vi "Core_Chem_User_Interface_v1.3.vi"() -> ()   [LabVIEW 2014]
uses:
  C:/Program Files (x86)/National Instruments/LabVIEW 2014/examples/Data Communication/Network Streams/Simple Network Streams/support/Network Stream Command.ctl
  <vilib>/dex/Stream Element Allocation Mode.ctl
  <vilib>/Platform/TimedLoop/XDataNode/wakeup.ctl
  <vilib>/Platform/TimedLoop/XDataNode/XDNodeRunTimeDep.lvlib
  <vilib>/Platform/TimedLoop/XDataNode/nitl_modes.ctl
  <vilib>/Platform/TimedLoop/XDataNode/timing_clust.ctl
  <vilib>/platform/TimedLoop/XDataNode/XDataNode.xnode
  <vilib>/Utility/tcp.llb/UDP Multicast Read-Only Open.vi
  <vilib>/FTP/NI_FTP.lvlib
panel:
  out "Create folder error out 2":errorcluster
  out "Network to cRIO live status":bool
  out "Create folder error out":errorcluster
  in  "Confirm Flight Number":bool
  out "PRTAFT_UDP_In":string
  out "TWBOZO01":string
  out "CABOZO01":string
  out "TEIOZO01":string
  out "CHTSOO01":string
  out "CHFGGA01":string
  out "AL52CO01":string
  in  "Flight Number":string
  in  "Tab Control":T1(tab)
  out "FGGA preflight Des 17":string="Preflight - Start minimum 2 hours before take-off\n\n1. Ensure no bags/jackets are stowed on seat backs and behind seats in front of core chemistry rack at all times.\n\n2. Remove inlet covers if applicable.\n\n3. Connect Lilliput mini TFT/LCD VGA cable to FGGA VIDEO (back panel) and PS2 Keyboard/Mouse cables to FGGA Connectors (back panel). TFT/LCD and Keyboard kept in Core Chemistry Dell laptop bag. Connect TFT/LCD AC/DC PSU to 6026-8-98 Amphenol (SSP9) and make 230 Vac CB.\n\n4. Ensure all circuit breakers are pushed in, except 230Vac and 28Vdc, UPS switch off (down) and AL5002 CO Plasma Lamp switch off (down).\n\n5. Wait for aircraft LAN to be up and running before start-up.\n\n6. Check AboutTime has synchronised laptop clock to aircraft timeservers (Filiberto/Gaston).\n\nClick the PowerUp Tab."
  out "FGGA preflight Des 16":string="PowerUp\n\n1.\tSSP9 forward face\tMake 3 CBs\n\n2.\tPWRDIST \t\tMake 230Vac CB Switch UPS On \t[UP]\n                     Make 28Vdc CB\n                     Check 28VDC OK Green Light comes on\n\n3.\tCore Chemistry e-Log\nComplete Core Chemistry e-Log in WordPad (Bnnn_CoreChemLog_v2.1), save on Flight Manager's laptop (192.168.101.180/      flt_folders/Bnnn); Fill in header with date, flight number and your name/initials.\n\n4.\tSAMPUMP\t\t\n - Switch WoW override key (vertical) to check pump starts, and MFM flowrate increase (>20 LPM) under System Overview tab. \n - Switch off WoW override\t\t\t\t [NORM, key horizontal]\n\nClick the 2B Ozone tab if operated, otherwise, click the UDP tab.\n\n\n"
  out "MFM":dbl(graph)
  in  "Ambient = OFF\nCabin = ON":bool
  out "FGGA preflight Des 15":string="2B Ozone Preflight\n\n1.\tSelect either Ambient or Cabin Air mode (default should be OFF for Ambient air mode).\n\n2. Check flowrate is greater than 2000 sccm.\n\nClick the UDP tab."
  out "2B Ozone concentration":dbl(graph)
  out "2B Ozone flow rate":dbl(graph)
  out "2BOzone Event error out":errorcluster
  out "2BOzone command sender error out":errorcluster
  out "FGGA preflight Des 14":string="UDP Preflight\n1. Check all UDP packets are updating.  Unix time increasing by 1 sec (2nd parameter).\n2. Check flight number is correct.\n3. Confirm flight number and check it appears in the UDP packet. "
  in  "name":string="239.1.4.6"
  in  "Port":u16=50001
  out "FGGA":string
  out "CO":string
  out "Ozone":string
  out "Cabin Ozone":string
  out "Ambient Ozone":string
  out "SO2":string
  out "Ozone Zeroing\nTime Remain (sec)":u32
  in  "Ozone Zeroing":bool
  out "TEI49C Sample Flow B":dbl(graph)
  out "TEi49C Concentration":dbl(graph)
  out "TEI49C Sample Flow A":dbl(graph)
  out "FGGA preflight Des 13":string="TEi49C Ozone PRE-FLIGHT - LAST ACTIONS BEFORE SEAT-BELTING DOWN (PRIOR TO ENGINES START)\n\n1. Ozone monitor zeroing\t\t[10 min minimum]\n\n\n2. Check TEi49C zero value and note down value in e-Log. \n"
  out "FGGA preflight Des 12":string="TEi49C Ozone Preflight\n\n1. Check nominal sample flowrate on both channels is ~0.7 LPM."
  out "Ozone Event error out":errorcluster
  out "Ozone command sender error out":errorcluster
  in  "Ozone UDP Time Offset":i32=1
  out "SO2 Flush\nTime Remain (sec)":u32
  out "TEI43i MFC3 Sample Flow":dbl(graph)
  out "TEi43C / TEi43i Concentration":dbl(graph)
  out "TEI43C Sample Flow":dbl(graph)
  out "TEI43i MFC2 Cal Flow":dbl(graph)
  in  "MFC_2 User Set Value":dbl=2.5
  in  "MFC_3 User Set Value":dbl=2.0
  out "SO2 CAL\nTime Remain (sec)":u32
  out "SO2 Cal Flush\nTime Remain (sec)":u32
  in  "SO2 CAL":bool
  out "FGGA preflight Des 11":string="TEi43 SO2 Inflight Calibration"
  in  "SO2 Zeroing":bool
  out "SO2 Zeroing\nTime Remain (sec)":u32
  out "FGGA preflight Des 10":string="TEi43 SO2 PRE-FLIGHT - LAST ACTIONS BEFORE SEAT-BELTING DOWN (PRIOR TO ENGINES START)\n\n1. SO2 monitors zeroing\t\t[10 min minimum]\n\n\n2. Check TEi43i or TEi43C zero value and note down value in e-Log. "
  in  "SO2 Flush":bool
  out "FGGA preflight Des 9":string="TEi43 SO2 Preflight\n\n1. Check nominal sample flowrate is 2.0 LPM.\n\nSO2 calibration gas purge - SO2 calibration cylinder locate at bottom of WAS Gas rack.\n\n2. Check quick connect male body is connected to 'chem 1' gas line.\n\n3. Open cylinder valve 1.\n\n4. Set regulator to deliver at 3 bar.\n\n5. Open regulator valve 3 (anti-clockwise).\n\n6. Close cylinder valve 1.\n\n7. Press SO2 flush button, MFC2 cal flow should increase to 2.5 SLPM.\nMonitor MFC2 flow rate to make sure the reading decreases from 2.5 SLPM to 0.0 SLPM.\nCheck pressure content and delivery guages also reasd zero.\nIf pressure content & delivery guages do NOT read zero, press SO2 flush button again until they do.\n\n8. Quickly open and close cylinder valve 1.\n\n9. Repeat step 7) to 8) three times.\n\n10. Open cylinder valve 1, system is ready.\n "
  in  "eV9 Flush User\nset time (sec)":i32=15
  in  "eV9 flush User\nset time (sec)":i32=60
  in  "eV8 User\nset time (sec)":i32=120
  out "SO2 Event error out":errorcluster
  out "SO2 command sender error out":errorcluster
  in  "SO2 UDP Time Offset":i32=1
  out "CO CAL Status":bool
  in  "CO CAL":bool
  out "FGGA preflight Des 8":string="CO Preflight and Inflight Calibrations\nHold down the CAL button for 2 secs then release, CAL status should then lit up"
  in  "Prepare Gases":bool
  out "FGGA preflight Des 7":string="AL5002 CO Preflight Checks\n\n1.\n\n2. Start CO Vacuum. NB: If there is problem with the software control, use manual override switch [up] on CALDECK front panel\n\n3. CO Checks - charts on the right hand side\n    Lamp Flow Controller ~ 40 ml/min\n    Monochromater Flow Controller ~ 30 ml/min\n    Fluorescence Cell Pressure ~ 7.5 Torr\n\nIf Lamp/Mono flows are low, manual valves (V1 -> V5) may still be shut, or pressure adjusting valves (ALREG1 & 2) have not been set > 2 bar\n\nIf Cell pressure is 10 Torr (max range), check that COPUMP is running and eV7 is opened (CALDECK green LED).\n\n4. Switch Plasma Lamp at the front panel UP\n\nDetector count rate (on 'Raw Signal' or F2 instrument touchscreen) should increase to >=10000 Hz within a minute.  Recycle plasma lamp switch (off/on) if no significant increase in count rate after 10 mins.  CO concentration should increase (100s ppb). \n     \n\n"
  in  "CO Vacuum (eV7)":bool
  out "Raw Signal":dbl(graph)
  out "CO Concentration":dbl(graph)
  out "Fluorsecence Cell Pressure":dbl(graph)
  out "Monochromater Flow":dbl(graph)
  out "Lamp Flow Controller":dbl(graph)
  in  "CO UDP Time Offset":i32=1
  out "CO2 Pressure\nDelivery (PSIA)":dbl(slide) scale=0.0..100.0
  out "Std\nContent (barG)":dbl(slide) scale=0.0..220.0
  out "N2\nContent (barG)":dbl(slide) scale=0.0..220.0
  out "CO2\nContent (barG)":dbl(slide) scale=0.0..170.0
  out "CO Event error out":errorcluster
  out "CO command sender error out":errorcluster
  out "CO Zero":T2(array[cluster])
  out "CO Sensitivity":T3(array[cluster])
  out "Cell temperature":dbl(graph)
  out "Cell pressure":dbl(graph)
  in  "Manual FGGA Pump":bool
  out "CO2":dbl(graph)
  out "CH4":dbl(graph)
  out "H2O":dbl(graph)
  out "WoW Flag":string="0"
  in  "FGGA pump\nsync to WoW":bool
  out "CH4 Dry":dbl(graph)
  out "CO2 Dry":dbl(graph)
  out "MFC1 Cal Flow":dbl(graph)
  out "Flush Target Tank\nTime Remain (sec)":u32
  out "Flush Low Tank\nTime Remain (sec)":u32
  out "Flush High Tank\nTime Remain (sec)":u32
  in  "Flush Target Tank":bool
  in  "Flush Low Tank":bool
  in  "Flush High Tank":bool
  in  "FGGA Restart":bool
  out "FGGA preflight Des 6":string="FGGA Instrument Controls"
  in  "High Cal":bool
  out "High Cal\nFlush Time Remain (sec)":u32
  out "High Cal\nCal Time Remain (sec)":u32
  in  "Low Cal":bool
  in  "Target Cal":bool
  in  "Span Cal - \nHigh Cal, CO Cal, Low Cal":bool
  out "Low Cal\nFlush Time Remain (sec)":u32
  out "Low Cal\nCal Time Remain (sec)":u32
  out "Target Cal\nFlush Time Remain (sec)":u32
  out "Target Cal\nCal Time Remain (sec)":u32
  in  "MFC_1 User Set Value":dbl=3.0
  out "FGGA preflight Des 5":string="FGGA Inflight Calibrations"
  out "FGGA preflight Des 4":string="FGGA Ground Preflight Checks\n\n1. Switch FGGA pump ON\n\n2. Check cavity pressure ~50 Torr\n\n3. Switch FGGA pump OFF\n\n4. Enable FGGA pump sync to WoW\n\n5.. Check Time Synchronisation\n\n6. Check CO2 & CH4 values\n"
  out "FGGA preflight Des 3":string="FGGA CAL Gas Purge\n\nFor each cylinder in gas stowage, check that,\n\n1. V1 Closed\n    V3 Closed\n    V4 Make sure arrow positioned downwards (i.e. flow points to gas line)\n\n2. V3 Open (turn anti-clockwise)\n\n3. Use the button on the right according to the operating cylinder to flush the line. Monitor the MFC flow rate to make sure the reading decreases from 3 to zero. (ie fully flushed). Pressure content & delivery gauges should also read zero.\n\n4. V3 Close (turn clockwise)\n\n5. V1 Open / Close quickly\n         Check delivery pressure gauge is ~ 40 PSI \n         (Use V2 to increase if necessary)\n\n6. Repeat steps 2) to 5) three times\n\n7. V3 Close (turn clockwise)\n\n8. V1 Open, check V2 ~ 40 PSIG\n\n9. V3 Open - System is ready"
  out "FGGA command sender error out":errorcluster
  out "FGGA Event Error out":errorcluster
  in  "FGGA UDP Time Offset":i32=1
  in  "FGGA Shutdown":bool
  in  "Postflight Procedures":bool
  in  "cRIO File IO Stop\n(USB Flash Drive Unmount)":bool
  in  "FTP ASCII Files to Local":bool
  in  "Transfer FGGA Files":bool
  out "FGGA preflight Des 18":string="Postflight\n\n1. Press the cRIO File IO Stop to stop ASCII file recording\nNote: ASCIII file recording will start again once the flight number is confirmed.\n\n2. Press the FTP ASCII File to Local button to transfer ASCII files to flight folder.\n\n\n3. Press the Transfer FGGA Files button to transfer FGGA files to flight folder. \n\n4. Shutdown FGGA.\n\n\n5. View Postflight Procedures."
  out "File List":string[](array[string])
  out "FGGA File Transfer Error out":errorcluster
  out "Move to FM Error out":errorcluster
  out "USB Disk Space Used %":dbl(slide) scale=0.0..100.0
  out "PTP Sync":bool
  out "CPU Total %":dbl(graph)
  out "PRTAFT_DLU":string
  in  "Inst_alm_thresh":i32=220
  in  "3hr_alm_thresh":i32=80
  in  "Simulate Inst Conc":i32
  in  "Simulate 3hr Average Conc":dbl
  in  "Simulate 2B Conc":bool
  in  "Ozone eV6":bool
  in  "Simulate Conc":bool
  in  "8hr TWA Limit":i32=490
  in  "10mins STEL Limit":i32=700
  in  "SO2 Slope":dbl=1.0
  in  "SO2 Offset":dbl
  in  "Simulate TWA Conc":dbl
  in  "Simulate STEL Conc":dbl
  in  "MFC_3\nSLPM Value":dbl=2.0
  in  "MFC_2\nSLPM Value":dbl
  in  "SO2 eV6":bool
  in  "eV8":bool
  in  "eV9":bool
  in  "eV4":bool
  in  "eV3":bool
  in  "MFC_1\nSLPM Value":dbl
  in  "eV2":bool
  in  "eV1":bool
  # "concentration\npmt_volt\nlamp_volt\nlamp_intens\ninternal_temper\nreact_temper\nreact_press\nflow\nflags\nten_min_so2\neight_hr_so2\nten_min_so2_alm\neight_hr_so2_alm\nMFC_2absolute_pres\nMFC_2temperature\nMFC_2volumetic_flow\nMFC_2mass_flow\nMFC_2set_point\nMFC_3_absolute_pres\nMFC_3_temperature\nMFC_3volumetic_flow\nMFC_3mass_flow\nMFC_3set_point\nV6\nV8\nV9\nMFC2_Set_Value\nMFC3_Set_Value"
  # "conc\ntemp\npress\nflow\nthreehr_oz\nInst_alarm\nthreehr_alarm"
  # "ch4\nco2\nh2o\npress_torr\ntemp_c\nfit_flag\nrda_usec\nrdb_usec\nch4_dry\nco2_dry\nMFC_1_absolute_pres\nMFC_1_temperature\nMFC_1volumetic_flow\nMFC_1mass_flow\nMFC_1set_point\nV1\nV2\nV3\nV4\nrestart_FGGA\nFGGA_Pump\nCAL_MFC_1Set_Value"
  # "conc\ntemp\npress\nflow"
  # "conc\nbenchtemp\npress\ncellAint\ncellBint\nFlowA\nFlowB\nlamptemp\nflag\nV6"
  # "conc\ncounts\nsens\nzero\nlampflow\nlamptemp\nmonoflow\nmonotemp\nmonopress\ncellpress\ncalpress\ntemppmt\ncalconc\nerr\ncal_counter\nerr_counter\nCO_vacuum_status\nIn_Cal\nALEG1_press_delivery\nALREG1_press_content\nALREG2_press_content\nALREG3_press_content"
  # "TEi43c"
  # "TEi43i"
  # "SO2 CAL SETTINGS"
  # "SO2 FLUSH SETTING"
  # "FGGA"
  # "2B Ozone"
  # "TEi49C  - Ozone"
  # "TEi43 - SO2"
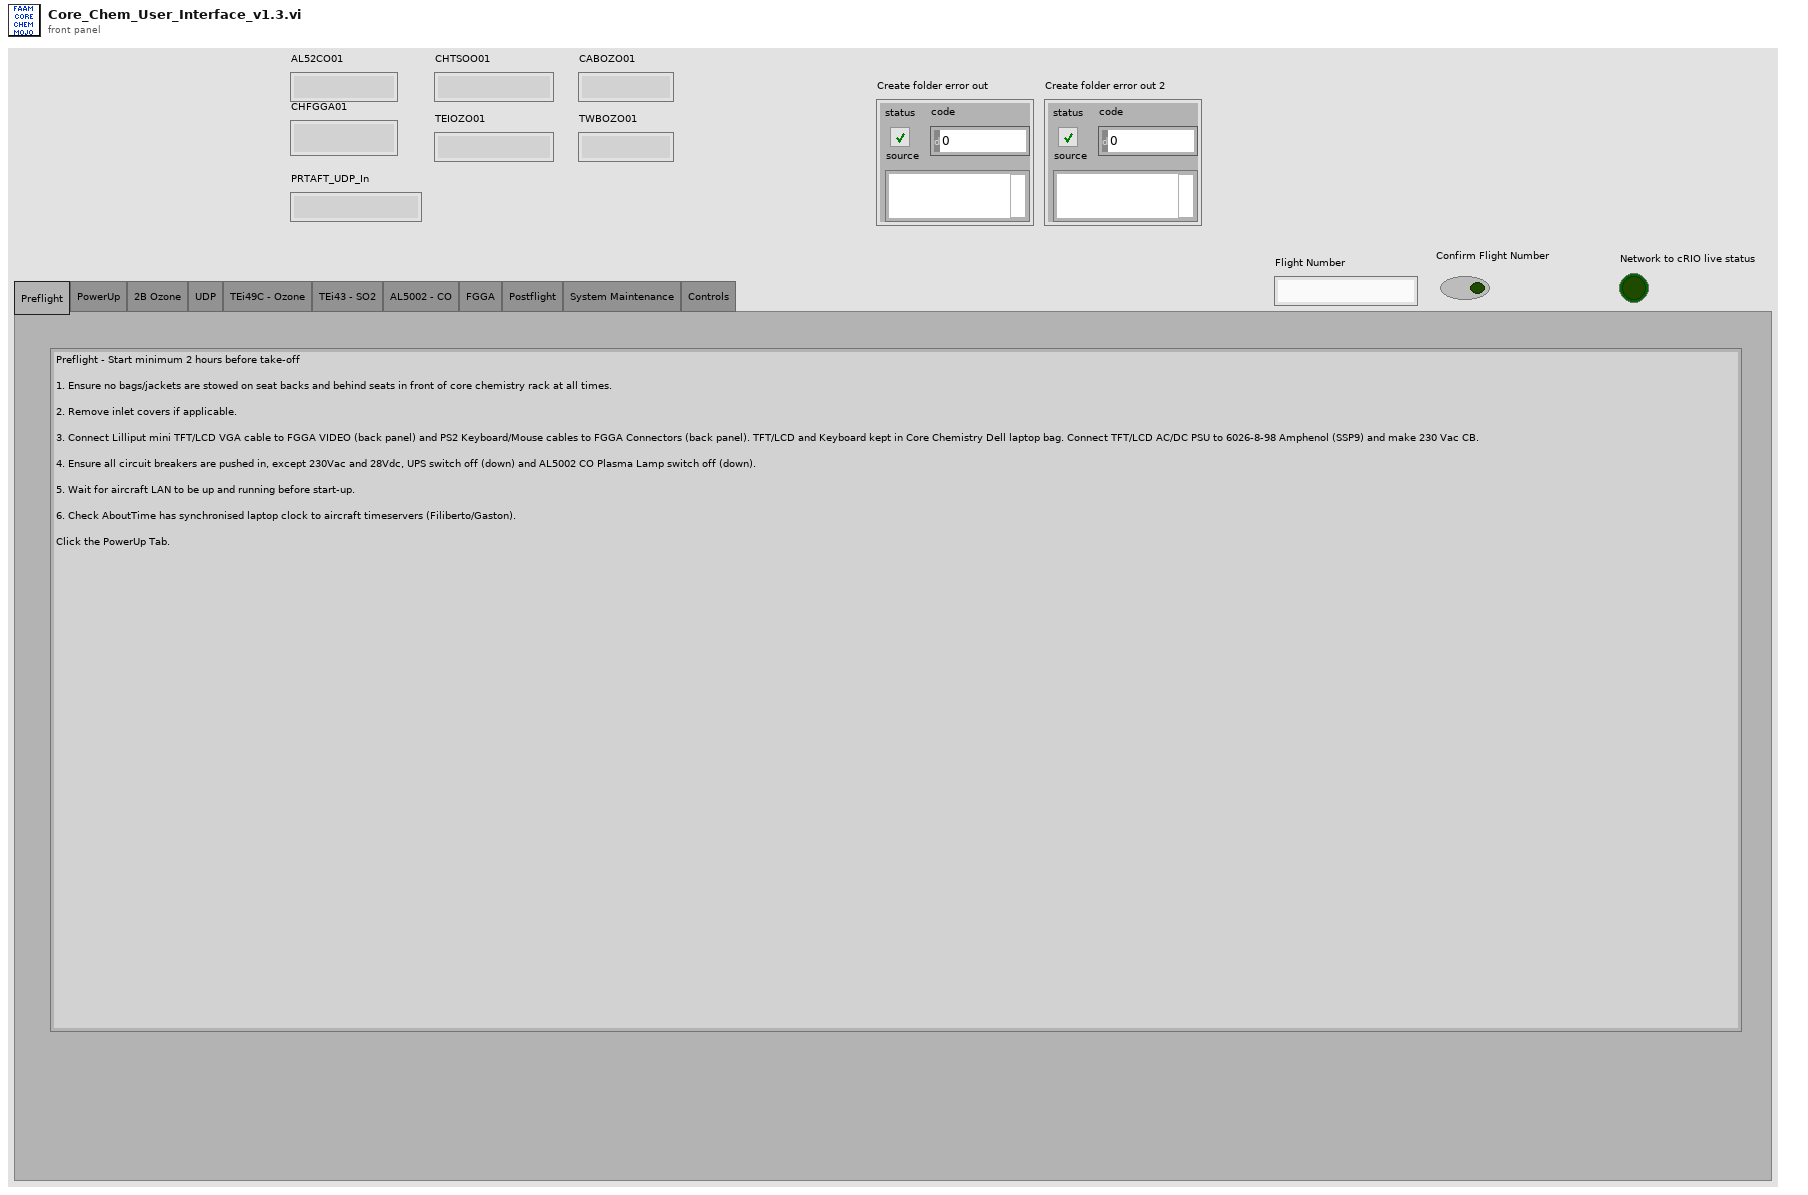
[diagram p1: front panel]
types:
  T1 = enum32{"Preflight", "PowerUp", "2B Ozone", "UDP", "TEi49C - Ozone", "TEi43 - SO2", "AL5002 - CO", "FGGA", "Postflight", "System Maintenance", "Controls"}
  T2 = cluster{"time stamp":timestamp, "CO Offset":dbl}[]
  T3 = cluster{"time stamp":timestamp, "CO Sensitivity":dbl}[]
  T4 = typedef "Network Stream Command.ctl" = cluster{"Message":string, "Message Data":variant}
  T5 = typedef "Stream Element Allocation Mode.ctl" = u32
  T6 = typedef "XDNodeRunTimeDep.lvlib/timing_clust.ctl" = cluster{"Expected End [f-1]":u64, "Actual End [f-1]":u64, "Finished Late? [f-1]":bool, "Expected End [i-1]":u64, "Actual End [i-1]":u64, "Finished Late? [i-1]":bool, "Expected Start [i]":u64, "Actual Start [i]":u64, "Expected Start [f]":u64, "Actual Start [f]":u64, "Source Name":string, "Structure Name":string, "Period":i64, "Deadline":i64, "Offset":i64, "Start":i64, "Priority":i32, "Timeout":i32, "Mode":T7, "Wakeup Reason":T8, "Error":errorcluster, "Source Type":string, "Secondary Source Type":string, "Global End Time":u64, "Global Start Time":u64, "Frame Duration":u64, "Iteration Duration":u64, "Assigned CPU":i32, "I/O Scan Engine Mode":u32}
  T7 = typedef "XDNodeRunTimeDep.lvlib/nitl_modes.ctl" = enum32{"No Change", "Process missed periods, maintain original phase", "Discard missed periods, maintain original phase", "Process missed periods, ignore original phase", "Discard missed periods, ignore original phase"}
  T8 = typedef "XDNodeRunTimeDep.lvlib/wakeup.ctl" = enum32{"Normal", "Aborted", "Asynchronous wakeup", "Timing source error", "Timed loop error", "Timeout"}
  T9 = typedef "NI_FTP.lvlib/FTP Session.ctl" = refnum<k5>
  T10 = typedef "NI_FTP.lvlib/FTP File Info.ctl" = cluster{"type":enum16{"unknown", "file", "dir", "link"}, "permissions":string, "owner":string, "group":string, "size":i32, "date":string, "name":string, "link name":string}
  T11 = cluster{"Message":string, "Message 2":string, "Message 3":string}
  T12 = cluster{"Message":string, "Message 2":string, "Message 3":string, "Message 4":string}
  T13 = cluster{"Message":string, "Message 3":string, "Message 4":string}
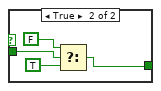
[diagram p10: hidden frame]
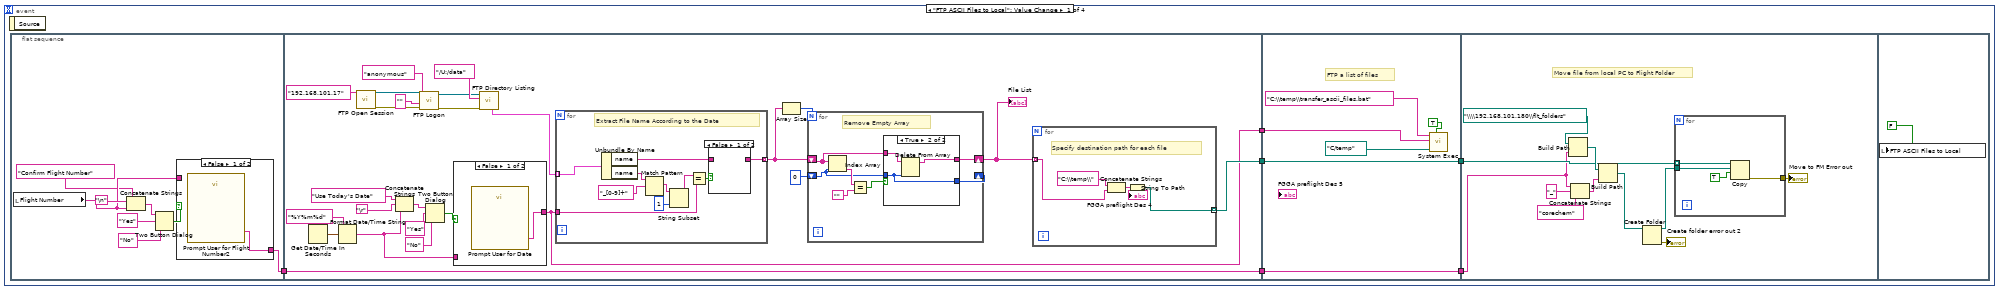
[diagram p13: hidden frame]
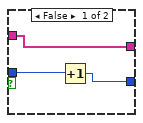
[diagram p16: hidden frame]
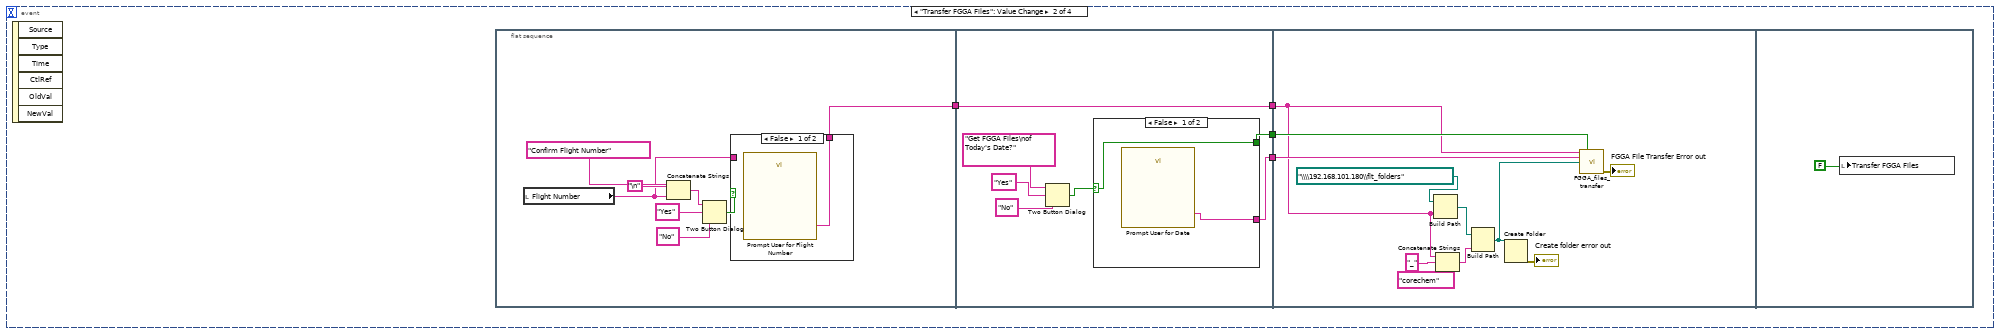
[diagram p18: hidden frame]
diagram:
  w4 = "XXXX"
  w7 = 0
  w8 = 0.0
  w14 = T4 {"Message"="", "Message Data"=variant} ("Message Cluster")
  w20 = T5 0 items=["allocate as needed", "pre-allocate"] ("element allocation mode")
  w26 = T4 {"Message"="", "Message Data"=variant} ("Message Cluster")
  w32 = T5 0 items=["allocate as needed", "pre-allocate"] ("element allocation mode")
  w37 = T4 {"Message"="", "Message Data"=variant} ("Message Cluster")
  w43 = T5 0 items=["allocate as needed", "pre-allocate"] ("element allocation mode")
  w53 = T5 0 items=["allocate as needed", "pre-allocate"] ("element allocation mode")
  w55 = T4 {"Message"="", "Message Data"=variant} ("Message Cluster")
  w62 = T5 0 items=["allocate as needed", "pre-allocate"] ("element allocation mode")
  w64 = T4 {"Message"="", "Message Data"=variant} ("Message Cluster")
  n1 = local write "cRIO File IO Stop\n(USB Flash Drive Unmount)"(FALSE ("Stop File Write")) -> ()
  n2 = local write "Flight Number"(w4) -> ()
  n3 = while {
    shift-right: [w68] -> _
    shift-left: w4 -> [w67]
    stop <- FALSE stop-if-true
    n4 = Not Equal?(x=w67, y="Flight Number") -> (x != y?=w70:bool)
    n5 = case shown="True" w70 {
      tunnel: [w73 w74] -> w68
      tunnel: "Flight Number" -> [_ w74]
      tunnel: w67 -> [w73 _]
      frame False {
      }
      frame True {
        n6 = One Button Dialog(message="Flight Number changed,\nPress flight number button to confirm") -> ()  [unwired: 1 in, 1 out]
      }
    }
    n7 = Wait (ms)(milliseconds to wait=u32 1000) -> ()  [unwired: 1 out]
  }
  n8 = while {
    stop <- FALSE stop-if-true
    # "UDP Read"
    n9 = String To IP(1:"name") -> (0:w81:u32)
    n10 = call-poly <vilib>:"UDP Multicast Open.vi"("multicast addr"=w81, "port"="Port") -> ("error out"=w79:errorcluster, "connection ID"=w78:refnum<k16>)  [unwired: 7 in, 1 out]
    n11 = Wait (ms)(milliseconds to wait=u32 1000) -> ()  [unwired: 1 out]
    n12 = case shown="No Error" w79 {
      selector: w79 -> [w85 _]
      tunnel: w78 -> [w84 _]
      frame No Error {
        w83 = ""
        n13 = while {
          tunnel: w85 -> [w131]
          tunnel: w84 -> [w130]
          shift-right: [w126] -> _
          shift-left: w83 -> [w127]
          shift-right: [w117] -> _
          shift-left: w83 -> [w119]
          shift-right: [w111] -> _
          shift-left: w83 -> [w113]
          shift-right: [w105] -> _
          shift-left: w83 -> [w106]
          shift-right: [w99] -> _
          shift-left: w83 -> [w100]
          shift-right: [w93] -> _
          shift-left: w83 -> [w94]
          shift-right: [w87] -> _
          shift-left: w83 -> [w88]
          stop <- w129 stop-if-true
          n14 = UDP Read(connection ID=w130, 8:w131) -> (data out=w86:string, error out=w129:errorcluster)  [unwired: 2 in, 3 out]
          n15 = Match Pattern(string=w86, regular expression="$TEIOZO01,") -> (match substring=w125:string, after substring=w124:string)  [unwired: 1 in, 2 out]
          n16 = Match Pattern(string=w86, regular expression="$TWBOZO01,") -> (match substring=w103:string, after substring=w102:string)  [unwired: 1 in, 2 out]
          n17 = Match Pattern(string=w86, regular expression="$CABOZO01,") -> (match substring=w109:string, after substring=w108:string)  [unwired: 1 in, 2 out]
          n18 = Match Pattern(string=w86, regular expression="$CHTSOO01,") -> (match substring=w97:string, after substring=w96:string)  [unwired: 1 in, 2 out]
          n19 = Match Pattern(string=w86, regular expression="$CHFGGA01,") -> (match substring=w121:string, after substring=w120:string)  [unwired: 1 in, 2 out]
          n20 = Match Pattern(string=w86, regular expression="$AL52CO01,") -> (match substring=w115:string, after substring=w114:string)  [unwired: 1 in, 2 out]
          n21 = Match Pattern(string=w86, regular expression="$PRTAFT01,") -> (match substring=w92:string, after substring=w91:string)  [unwired: 1 in, 2 out]
          n22 = Concatenate Strings(w125, w124) -> (w123:string)
          n23 = Concatenate Strings(w103, w102) -> (w101:string)
          n24 = Concatenate Strings(w109, w108) -> (w107:string)
          n25 = Concatenate Strings(w97, w96) -> (w95:string)
          n26 = Concatenate Strings(w121, w120) -> (w118:string)
          n27 = Concatenate Strings(w115, w114) -> (w112:string)
          n28 = Concatenate Strings(w92, w91) -> (w89:string)
          n29 = Replace Substring(4:w101, 5:w100) -> (1:w99:string)  [unwired: 2 in, 1 out]
          "TWBOZO01" <- w99
          n30 = Replace Substring(4:w123, 5:w127) -> (1:w126:string)  [unwired: 2 in, 1 out]
          "TEIOZO01" <- w126
          n31 = Replace Substring(4:w107, 5:w106) -> (1:w105:string)  [unwired: 2 in, 1 out]
          "CABOZO01" <- w105
          n32 = Replace Substring(4:w95, 5:w94) -> (1:w93:string)  [unwired: 2 in, 1 out]
          "CHTSOO01" <- w93
          n33 = Replace Substring(4:w112, 5:w113) -> (1:w111:string)  [unwired: 2 in, 1 out]
          "AL52CO01" <- w111
          n34 = Replace Substring(4:w118, 5:w119) -> (1:w117:string)  [unwired: 2 in, 1 out]
          "CHFGGA01" <- w117
          n35 = Replace Substring(4:w89, 5:w88) -> (1:w87:string)  [unwired: 2 in, 1 out]
          "PRTAFT_UDP_In" <- w87
        }
      }
      frame Error {
      }
    }
  }
  n36 = Obtain Queue(name (unnamed)="CO_Command", element data type=w64) -> (queue out=w13:refnum<queue>, error out=w58:errorcluster)  [unwired: 3 in, 1 out]
  n37 = Create Network Stream Writer Endpoint(6:w62, 7:10 ("writer buffer size"), 9:w64, 10:"//192.168.101.17/command/reader/CO" ("reader url"), 11:"/command/writer/CO" ("writer name")) -> (0:w61:errorcluster, 3:w60:refnum<k21>)  [unwired: 2 in]
  n38 = while {
    tunnel: w13 -> [w135]
    tunnel: w58 -> [w134]
    tunnel: [w132] -> _
    stop <- FALSE stop-if-true
    # "CO UI Event Handler Loop"
    n39 = event shown="[4] \"Confirm Flight Number\": Value Change" {
      selector: _ -> [_ _ _ _ _]
      dyn-events: _ -> [_ _ _ _ _]
      timeout: _ -> [_ _ _ _ _]
      tunnel: w135 -> [w142 w149 w153 w160 w167]
      tunnel: w134 -> [w141 w148 w152 w159 w166]
      tunnel: [w136 w143 w151 w158 w165] -> w132
      event "CO CAL": Value Change {
        n40 = event-data() -> ("NewVal"=w139:bool)  [unwired: 1 in]
        n41 = Bundle(cluster=T4 {"Message"="", "Message Data"=variant} ("Message Cluster"), "Message"="CO CAL", "Message Data"=w139) -> (w137:T4)
        n42 = Enqueue Element(queue=w142, element=w137, error in (no error)=w141) -> (error out=w136:errorcluster)  [unwired: 1 in, 2 out]
      }
      event "CO UDP Time Offset": Value Change {
        n43 = event-data() -> ("NewVal"=w146:i32)  [unwired: 1 in]
        n44 = Bundle(cluster=T4 {"Message"="", "Message Data"=variant} ("Message Cluster"), "Message"="UDP Time Offset", "Message Data"=w146) -> (w144:T4)
        n45 = Enqueue Element(queue=w149, element=w144, error in (no error)=w148) -> (error out=w143:errorcluster)  [unwired: 1 in, 2 out]
      }
      event "CO Vacuum (eV7)": Value Change {
        n46 = event-data() -> ("NewVal"=w150:bool)  [unwired: 1 in]
        n47 = Bundle(cluster=T4 {"Message"="", "Message Data"=variant} ("Message Cluster"), "Message"="CO Vacuum", "Message Data"=w150) -> (w154:T4)
        n48 = Enqueue Element(queue=w153, element=w154, error in (no error)=w152) -> (error out=w151:errorcluster)  [unwired: 1 in, 2 out]
      }
      event "cRIO File IO Stop\n(USB Flash Drive Unmount)": Value Change {
        n49 = event-data() -> ("NewVal"=w157:bool)  [unwired: 1 in]
        n50 = Bundle(cluster=T4 {"Message"="", "Message Data"=variant} ("Message Cluster"), "Message"="Stop File Write", "Message Data"=w157) -> (w161:T4)
        n51 = Enqueue Element(queue=w160, element=w161, error in (no error)=w159) -> (error out=w158:errorcluster)  [unwired: 1 in, 2 out]
      }
      event "Confirm Flight Number": Value Change {
        n52 = event-data() -> ()  [unwired: 1 in, 1 out]
        n53 = local read "Flight Number"() -> (w164:string)
        n54 = Bundle(cluster=T4 {"Message"="", "Message Data"=variant} ("Message Cluster"), "Message"="Flight Number", "Message Data"=w164) -> (w168:T4)
        n55 = Enqueue Element(queue=w167, element=w168, error in (no error)=w166) -> (error out=w165:errorcluster)  [unwired: 1 in, 2 out]
      }
    }
    "CO Event error out" <- w132
  }
  n56 = while {
    tunnel: w13 -> [w178]
    shift-right: [w173] -> _
    shift-left: w60 -> [w175]
    shift-right: [w171] -> w49
    shift-left: w61 -> [w177]
    tunnel: w58 -> [w172]
    stop <- w171 stop-if-true
    # "CO UI Command Sender"
    n57 = Dequeue Element(queue=w178, error in (no error)=w172) -> (element=w174:T4)  [unwired: 1 in, 3 out]
    n58 = Unbundle By Name(w174) -> ("Message"=w176:string)
    n59 = case shown="\"UDP Time Offset\"" w176 {
      tunnel: w177 -> [w179 w183 w190 w197 w204 w211]
      tunnel: w175 -> [w180 w186 w193 w200 w207 w214]
      tunnel: w174 -> [_ w185 w192 w199 w206 w213]
      tunnel: [w179 w182 w189 w196 w203 w210] -> w171
      tunnel: [w180 w181 w188 w195 w202 w209] -> w173
      frame "False", Default {
      }
      frame "CO CAL" {
        n60 = shared-variable-write(w186, w183, w185) -> (w184:refnum<k21>, w187:errorcluster)  [unwired: 1 in, 1 out]
        n61 = Flush Stream(8:w187, 11:w184) -> (0:w182:errorcluster, 3:w181:refnum<k21>)  [unwired: 2 in, 1 out]
      }
      frame "UDP Time Offset" {
        n62 = shared-variable-write(w193, w190, w192) -> (w191:refnum<k21>, w194:errorcluster)  [unwired: 1 in, 1 out]
        n63 = Flush Stream(8:w194, 11:w191) -> (0:w189:errorcluster, 3:w188:refnum<k21>)  [unwired: 2 in, 1 out]
      }
      frame "Stop File Write" {
        n64 = shared-variable-write(w200, w197, w199) -> (w198:refnum<k21>, w201:errorcluster)  [unwired: 1 in, 1 out]
        n65 = Flush Stream(8:w201, 11:w198) -> (0:w196:errorcluster, 3:w195:refnum<k21>)  [unwired: 2 in, 1 out]
      }
      frame "Flight Number" {
        n66 = shared-variable-write(w207, w204, w206) -> (w205:refnum<k21>, w208:errorcluster)  [unwired: 1 in, 1 out]
        n67 = Flush Stream(8:w208, 11:w205) -> (0:w203:errorcluster, 3:w202:refnum<k21>)  [unwired: 2 in, 1 out]
      }
      frame "CO Vacuum" {
        n68 = shared-variable-write(w214, w211, w213) -> (w212:refnum<k21>, w215:errorcluster)  [unwired: 1 in, 1 out]
        n69 = Flush Stream(8:w215, 11:w212) -> (0:w210:errorcluster, 3:w209:refnum<k21>)  [unwired: 2 in, 1 out]
      }
    }
  }
  "CO command sender error out" <- w49
  n70 = node-c288() -> (w12:T6)  [unwired: 4 in]
  n71 = Initialize Array(cluster{"time stamp":timestamp, "Y":dbl} {"time stamp"=timestamp(0 s since 1904-01-01), "Y"=0.0}, 30 ("dimension size")) -> (w9:cluster{"time stamp":timestamp, "Y":dbl}[])
  n72 = timed-loop {
    timing: w12 -> [_]
    timing-out: [_] -> w11
    stop <- _ stop-if-true
    # "PC Tasks"
    n73 = node-c288() -> ()  [unwired: 1 in, 1 out]
    n74 = event shown="[2] \"FGGA Restart\": Value Change" {
      selector: _ -> [_ _ _ _]
      dyn-events: _ -> [_ _ _ _]
      timeout: _ -> [_ _ _ _]
      event "FTP ASCII Files to Local": Value Change {
        n75 = event-data() -> ()  [unwired: 1 in, 1 out]
        n76 = flat-sequence {
          tunnel: [w224] -> w218
          tunnel: [w236] -> w223
          tunnel: [w235] -> w221
          tunnel: [w234] -> w219
          tunnel: w218 -> [w234]
          tunnel: w223 -> [w294]
          tunnel: [w294] -> w222
          tunnel: w221 -> [w290]
          tunnel: [w289] -> w220
          tunnel: w219 -> [w289]
          tunnel: w222 -> [w300]
          tunnel: w220 -> [w295]
          frame #0 {
            n77 = local read "Flight Number"() -> (w226:string)
            n78 = Concatenate Strings("Confirm Flight Number" ("message"), "\n", w226) -> (w230:string)
            n79 = Two Button Dialog(message=w230, 1:"No" ("F button name (\"Cancel\")"), 2:"Yes" ("T button name (\"OK\")")) -> (T button?=w227:bool)
            n80 = case shown="False" w227 {
              tunnel: w226 -> [_ w233]
              tunnel: [w232 w233] -> w224
              frame False {
                n81 = call "Prompt User for Flight Number2"() -> ("Flight Number BXXX"=w232:string)  [unwired: 17 in, 2 out]
              }
              frame True {
              }
            }
          }
          frame #1 {
            n82 = Get Date/Time In Seconds() -> (seconds since 1Jan1904=w240:timestamp)
            n83 = Format Date/Time String(time format string (%c)="%Y%m%d", seconds (now)=w240) -> (date/time string=w238:string)  [unwired: 1 in]
            n84 = call <vilib>:"FTP Open Session.vi"("address"="192.168.101.17") -> ("error out"=w255:errorcluster, "ftp session"=w256:T9)  [unwired: 7 in, 2 out]
            n85 = Concatenate Strings("Use Today's Date" ("message"), "\r", w238) -> (w244:string)
            n86 = call <vilib>:"FTP Logon.vi"("error in (no error)"=w255, "password"="", "user"="anonymous", "ftp session"=w256) -> ("error out"=w252:errorcluster, "ftp session out"=w251:T9)  [unwired: 4 in, 2 out]
            n87 = Two Button Dialog(message=w244, 1:"No" ("F button name (\"Cancel\")"), 2:"Yes" ("T button name (\"OK\")")) -> (T button?=w241:bool)
            n88 = case shown="False" w241 {
              tunnel: [w259 w260] -> w235
              tunnel: w238 -> [_ w260]
              frame False {
                n89 = call "Prompt User for Date"() -> ("Date"=w259:string)  [unwired: 17 in, 2 out]
              }
              frame True {
              }
            }
            n90 = call <vilib>:"FTP Directory Listing.vi"("error in (no error)"=w252, "directory path"="/U:/data", "ftp session"=w251) -> ("dir list"=w250:T10[])  [unwired: 4 in, 4 out]
            n91 = for {
              tunnel: w250 -> [w280] mode=indexing
              tunnel: [w279] -> w247 mode=indexing
              tunnel: w235 -> [w278]
              # "Extract File Name According to the Date"
              n92 = Unbundle By Name(w280) -> ("name"=w286:string, "name"=w285:string)
              n93 = Match Pattern(string=w285, regular expression="_[0-9]+") -> (match substring=w283:string)  [unwired: 1 in, 3 out]
              n94 = String Subset(string=w283, offset (0)=1) -> (substring=w281:string)  [unwired: 1 in]
              n95 = Equal?(x=w281, y=w278) -> (x = y?=w287:bool)
              n96 = case shown="False" w287 {
                tunnel: w286 -> [_ w288]
                tunnel: [_ w288] -> w279
                frame False {
                }
                frame True {
                }
              }
            }
            n97 = Array Size(array=w247) -> (size(s)=w249:i32)
            n98 = for {
              N: w249 -> [_]
              shift-right: [w267] -> w237
              shift-left: w247 -> [w268]
              shift-right: [w265] -> _
              shift-left: 0 -> [w266]
              # "Remove Empty Array"
              n99 = Index Array(array=w268, index=w266) -> (element=w270:string)
              n100 = Equal?(x=w270, y="") -> (x = y?=w269:bool)
              n101 = case shown="True" w269 {
                tunnel: w268 -> [w274 w277]
                tunnel: w266 -> [w273 w275]
                tunnel: [w274 w276] -> w267
                tunnel: [w272 w275] -> w265
                frame False {
                  n102 = Increment(x=w273) -> (x+1=w272:i32)
                }
                frame True {
                  n103 = Delete From Array(array=w277, index=w275) -> (array with subset deleted=w276:string[])  [unwired: 1 in, 1 out]
                }
              }
            }
            "File List" <- w237
            n104 = for {
              tunnel: w237 -> [w263] mode=indexing
              tunnel: [w261] -> w236 mode=indexing
              # "Specify destination path for each file"
              n105 = Concatenate Strings("C:\\temp\\", w263) -> (w262:string)
              n106 = String To Path(string=w262) -> (path=w261:path)
            }
          }
          frame #2 {
            # "FTP a list of files"
            n107 = call <vilib>:"System Exec.vi"("wait until completion? (T)"=TRUE, "working directory"=path "C:/temp", "standard input"=w290, "command line"="C:\\temp\\transfer_ascii_files.bat") -> ()  [unwired: 4 in, 4 out]
          }
          frame #3 {
            # "Move file from local PC to Flight Folder"
            n108 = Build Path(base path=path "\\\\192.168.101.180\\flt_folders" ("path"), name or relative path=w295) -> (appended path=w302:path)
            n109 = Concatenate Strings(w295, "_" ("string"), "corechem" ("string")) -> (w301:string)
            n110 = Build Path(base path=w302, name or relative path=w301) -> (appended path=w297:path)
            n111 = Create Folder(path (use dialog)=w297) -> (created path=w296:path, error out=→"Create folder error out 2":errorcluster)  [unwired: 2 in, 1 out]
            n112 = for {
              tunnel: w296 -> [w309]
              tunnel: [w308] -> w299
              tunnel: w300 -> [w306] mode=indexing
              n113 = Copy(9:TRUE ("overwrite (F)"), 10:w309, 11:w306) -> (0:w308:errorcluster)  [unwired: 2 in, 2 out]
            }
            "Move to FM Error out" <- w299
          }
          frame #4 {
            n114 = local write "FTP ASCII Files to Local"(FALSE ("FTP Files to Local")) -> ()
          }
        }
      }
      event "Transfer FGGA Files": Value Change {
        n115 = event-data() -> ()  [unwired: 1 in, 6 out]
        n116 = flat-sequence {
          tunnel: [w315] -> w314
          tunnel: w314 -> [w327]
          tunnel: [w327] -> w313
          tunnel: [w326] -> w312
          tunnel: [w325] -> w311
          tunnel: w313 -> [w343]
          tunnel: w312 -> [w345]
          tunnel: w311 -> [w344]
          frame #0 {
            n117 = local read "Flight Number"() -> (w316:string)
            n118 = Concatenate Strings("Confirm Flight Number" ("message"), "\n", w316) -> (w318:string)
            n119 = Two Button Dialog(message=w318, 1:"No" ("F button name (\"Cancel\")"), 2:"Yes" ("T button name (\"OK\")")) -> (T button?=w322:bool)
            n120 = case shown="False" w322 {
              tunnel: w316 -> [_ w324]
              tunnel: [w323 w324] -> w315
              frame False {
                n121 = call "Prompt User for Flight Number"() -> ("Flight Number BXXX"=w323:string)  [unwired: 17 in, 2 out]
              }
              frame True {
              }
            }
          }
          frame #1 {
            n122 = Two Button Dialog(message="Get FGGA Files\nof Today's Date?", 1:"No" ("F button name (\"Cancel\")"), 2:"Yes" ("T button name (\"OK\")")) -> (T button?=w331:bool)
            n123 = case shown="False" w331 {
              selector: w331 -> [w333 w334]
              tunnel: [w333 w334] -> w325
              tunnel: [w332 _] -> w326
              frame False {
                n124 = call "Prompt User for Date"() -> ("Date"=w332:string)  [unwired: 17 in, 2 out]
              }
              frame True {
              }
            }
          }
          frame #2 {
            n125 = Build Path(base path=path "\\\\192.168.101.180\\flt_folders" ("path"), name or relative path=w343) -> (appended path=w337:path)
            n126 = Concatenate Strings(w343, "_" ("string"), "corechem" ("string")) -> (w336:string)
            n127 = Build Path(base path=w337, name or relative path=w336) -> (appended path=w342:path)
            n128 = Create Folder(path (use dialog)=w342) -> (error out=→"Create folder error out":errorcluster)  [unwired: 2 in, 2 out]
            n129 = call "FGGA_files_transfer.vi"("Flight_num"=w343, "Get current?"=w344, "Date"=w345, "Flight Folder Path"=w342) -> ("error IO"=→"FGGA File Transfer Error out":errorcluster)  [unwired: 11 in]
          }
          frame #3 {
            n130 = local write "Transfer FGGA Files"(FALSE) -> ()
          }
        }
      }
      event "FGGA Restart": Value Change {
        n131 = event-data() -> ()  [unwired: 1 in, 6 out]
        n132 = flat-sequence {
          frame #0 {
            n133 = Two Button Dialog(message="FGGA will be restarted,\nARE YOU SURE?") -> (T button?=w348:bool)  [unwired: 2 in]
            n134 = case shown="True" w348 {
              frame False {
              }
              frame True {
                n135 = call <vilib>:"System Exec.vi"("working directory"=path "C:/temp", "command line"="C:\\temp\\restart_fgga.bat") -> ()  [unwired: 6 in, 4 out]
              }
            }
          }
          frame #1 {
            n136 = local write "FGGA Restart"(FALSE ("FGGA Restart")) -> ()
          }
        }
      }
      event "FGGA Shutdown": Value Change {
        n137 = event-data() -> ()  [unwired: 1 in, 6 out]
        n138 = flat-sequence {
          frame #0 {
            n139 = Two Button Dialog(message="FGGA will be shutdown,\nARE YOU SURE?") -> (T button?=w353:bool)  [unwired: 2 in]
            n140 = case shown="True" w353 {
              frame False {
              }
              frame True {
                n141 = call <vilib>:"System Exec.vi"("working directory"=path "C:/temp", "command line"="C:\\temp\\shutdown_fgga.bat") -> ()  [unwired: 6 in, 4 out]
              }
            }
          }
          frame #1 {
            n142 = local write "FGGA Shutdown"(FALSE ("FGGA Restart")) -> ()
          }
        }
      }
    }
    n143 = node-c288() -> ()  [unwired: 1 in, 1 out]
  }
  n144 = while {
    shift-right: [w440] -> _
    shift-left: w8 -> [w438]
    shift-right: [w442] -> _
    shift-left: w7 -> [w443]
    shift-right: [w441] -> _
    shift-left: w9 -> [w445]
    shift-right: [w433] -> _
    shift-left: w9 -> [w435]
    shift-right: [w430] -> _
    shift-left: w8 -> [w429]
    shift-right: [w432] -> _
    shift-left: w7 -> [w434]
    shift-right: [w425] -> _
    shift-left: FALSE -> [w426]
    stop <- FALSE stop-if-true
    w372 = ""
    w367 = "%s" ("format string")
    w564 = "%s" ("format string")
    w569 = "%s" ("format string")
    w574 = "%s" ("format string")
    w580 = "%s" ("format string")
    w586 = "%s" ("format string")
    w590 = "%s" ("format string")
    # "UDP Data Processing"
    n145 = local read "CHFGGA01"() -> (w593:string)
    n146 = local read "TWBOZO01"() -> (w568:string)
    n147 = local read "AL52CO01"() -> (w585:string)
    n148 = local read "CABOZO01"() -> (w573:string)
    n149 = local read "TEIOZO01"() -> (w579:string)
    n150 = local read "CHTSOO01"() -> (w563:string)
    n151 = local read "PRTAFT_UDP_In"() -> (w365:string)
    n152 = local read "Ambient = OFF\nCabin = ON"() -> (w467:bool)
    n153 = Spreadsheet String To Array(delimiter (Tab)=",", format string=w590, spreadsheet string=w593, array type (2D Dbl)=string[] []) -> (array=w540:string[])
    n154 = Spreadsheet String To Array(delimiter (Tab)=",", format string=w586, spreadsheet string=w585, array type (2D Dbl)=string[] []) -> (array=w561:string[])
    n155 = Spreadsheet String To Array(delimiter (Tab)=",", format string=w574, spreadsheet string=w573, array type (2D Dbl)=string[] []) -> (array=w464:string[])
    n156 = Spreadsheet String To Array(delimiter (Tab)=",", format string=w580, spreadsheet string=w579, array type (2D Dbl)=string[] []) -> (array=w538:string[])
    n157 = Spreadsheet String To Array(delimiter (Tab)=",", format string=w569, spreadsheet string=w568, array type (2D Dbl)=string[] []) -> (array=w463:string[])
    n158 = Spreadsheet String To Array(delimiter (Tab)=",", format string=w564, spreadsheet string=w563, array type (2D Dbl)=string[] []) -> (array=w536:string[])
    n159 = Array To Spreadsheet String(delimiter (Tab)="\r", array=w540, 3:w590) -> (spreadsheet string=→"FGGA":string)
    n160 = Array To Spreadsheet String(delimiter (Tab)="\r", array=w561, 3:w586) -> (spreadsheet string=→"CO":string)
    n161 = Array To Spreadsheet String(delimiter (Tab)="\r", array=w464, 3:w574) -> (spreadsheet string=→"Cabin Ozone":string)
    n162 = Array To Spreadsheet String(delimiter (Tab)="\r", array=w538, 3:w580) -> (spreadsheet string=→"Ozone":string)
    n163 = Spreadsheet String To Array(delimiter (Tab)=",", format string=w367, spreadsheet string=w365, array type (2D Dbl)=string[] []) -> (array=w366:string[])
    n164 = Array To Spreadsheet String(delimiter (Tab)="\r", array=w463, 3:w569) -> (spreadsheet string=→"Ambient Ozone":string)
    n165 = Array To Spreadsheet String(delimiter (Tab)="\r", array=w536, 3:w564) -> (spreadsheet string=→"SO2":string)
    n166 = Array To Spreadsheet String(delimiter (Tab)="\r", array=w366, 3:w367) -> (spreadsheet string=→"PRTAFT_DLU":string)
    n167 = Index Array(array=w366, index #1=5 ("index"), index #2=19 ("index")) -> (element #1=w370:string, element #2=w368:string)
    n168 = Select(t=w464, s=w467, f=w463) -> (s? t:f=w462:string[])
    n169 = Not Equal?(x=w370, y=w372) -> (x != y?=w371:bool)
    n170 = Not Equal?(x=w368, y=w372) -> (x != y?=w369:bool)
    n171 = Index Array(array=w536, index #1=6 ("index"), index #2=4 ("index"), index #3=3 ("index"), index #4=7 ("index"), index #5=8 ("index"), index #6=15 ("index"), index #7=24 ("index"), index #8=29 ("index")) -> (element #1=w453:string, element #2=w519:string, element #3=w514:string, element #4=w507:string, element #5=w483:string, element #6=w482:string, element #7=w390:string, element #8=w389:string)
    n172 = Index Array(array=w462, index #1=8 ("index"), index #2=11 ("index")) -> (element #1=w456:string, element #2=w457:string)
    n173 = Index Array(array=w538, index #1=6 ("index"), index #2=4 ("index"), index #3=3 ("index"), index #4=7 ("index"), index #5=9 ("index"), index #6=14 ("index"), index #7=15 ("index")) -> (element #1=w532:string, element #2=w520:string, element #3=w515:string, element #4=w500:string, element #5=w473:string, element #6=w472:string, element #7=w471:string)
    n174 = case shown="False" w369 {
      tunnel: ["1" w599] -> w362
      tunnel: w368 -> [_ w599]
      frame False {
      }
      frame True {
      }
    }
    n175 = case shown="False" w371 {
      tunnel: ["XXXX" w601] -> w363
      tunnel: w370 -> [_ w601]
      frame False {
      }
      frame True {
      }
    }
    n176 = Scan Value(string=w456, format string="%f") -> (value=→"2B Ozone concentration":dbl)  [unwired: 1 in, 1 out]
    n177 = Scan Value(string=w457, format string="%f") -> (value=→"2B Ozone flow rate":dbl)  [unwired: 1 in, 1 out]
    n178 = Scan Value(string=w390, format string="%f") -> (value=→"TEI43i MFC2 Cal Flow":dbl)  [unwired: 1 in, 1 out]
    n179 = Scan Value(string=w389, format string="%f") -> (value=→"TEI43i MFC3 Sample Flow":dbl)  [unwired: 1 in, 1 out]
    n180 = Scan Value(string=w483, format string="%f") -> (value=→"TEi43C / TEi43i Concentration":dbl)  [unwired: 1 in, 1 out]
    n181 = Scan Value(string=w482, format string="%f") -> (value=→"TEI43C Sample Flow":dbl)  [unwired: 1 in, 1 out]
    n182 = Index Array(array=w540, index #1=6 ("index"), index #2=4 ("index"), index #3=3 ("index"), index #4=7 ("index"), index #5=8 ("index"), index #6=9 ("index"), index #7=10 ("index"), index #8=17 ("index"), index #9=16 ("index"), index #10=11 ("index"), index #11=12 ("index"), index #12=21 ("index")) -> (element #1=w534:string, element #2=w522:string, element #3=w517:string, element #4=w502:string, element #5=w414:string, element #6=w411:string, element #7=w406:string, element #8=w404:string, element #9=w401:string, element #10=w396:string, element #11=w395:string, element #12=w382:string)
    n183 = local write "WoW Flag"(w362) -> ()
    n184 = local write "Flight Number"(w363) -> ()
    n185 = Index Array(array=w561, index #1=2 ("index"), index #2=27 ("index"), index #3=28 ("index"), index #4=29 ("index"), index #5=30 ("index"), index #6=31 ("index"), index #7=6 ("index"), index #8=4 ("index"), index #9=3 ("index"), index #10=8 ("index"), index #11=14 ("index"), index #12=16 ("index"), index #13=19 ("index"), index #14=12 ("index"), index #15=13 ("index"), index #16=10 ("index"), index #17=11 ("index")) -> (element #1=w424:string, element #2=w504:string, element #3=w551:string, element #4=w545:string, element #5=w543:string, element #6=w544:string, element #7=w533:string, element #8=w521:string, element #9=w516:string, element #10=w505:string, element #11=w492:string, element #12=w489:string, element #13=w488:string, element #14=w448:string, element #15=w447:string, element #16=w378:string, element #17=w359:string)
    n186 = Decimal String To Number(string=w424) -> (number=w422:i32)  [unwired: 2 in, 1 out]
    n187 = call "Find_Data_SubVI.vi"("FGGA"=w534, "CO"=w533, "Ozone"=w532, "SO2"=w453) -> ("Output Value"=→"CPU Total %":dbl)  [unwired: 11 in]
    n188 = call "Find_Data_SubVI.vi"("FGGA"=w522, "CO"=w521, "Ozone"=w520, "SO2"=w519) -> ("Output Value"=→"MFM":dbl)  [unwired: 11 in]
    n189 = call "Find_Data_SubVI.vi"("FGGA"=w517, "CO"=w516, "Ozone"=w515, "SO2"=w514) -> ("Output Value"=w513:dbl)  [unwired: 11 in]
    n190 = call "Find_Data_SubVI.vi"("FGGA"=w502, "CO"=w505, "Ozone"=w500, "SO2"=w507) -> ("Output Value"=→"USB Disk Space Used %":dbl)  [unwired: 11 in]
    n191 = Not Equal To 0?(x=w513) -> (x != 0?=→"PTP Sync":bool)
    n192 = Add(x=w422, y=u32 2082844800) -> (x+y=w421:u32)
    n193 = Scan Value(string=w382, format string="%f") -> (value=→"MFC1 Cal Flow":dbl)  [unwired: 1 in, 1 out]
    n194 = Scan Value(string=w395, format string="%f") -> (value=→"Cell temperature":dbl)  [unwired: 1 in, 1 out]
    n195 = Scan Value(string=w396, format string="%f") -> (value=→"Cell pressure":dbl)  [unwired: 1 in, 1 out]
    n196 = Scan Value(string=w401, format string="%f") -> (value=→"CH4 Dry":dbl)  [unwired: 1 in, 1 out]
    n197 = Scan Value(string=w404, format string="%f") -> (value=→"CO2 Dry":dbl)  [unwired: 1 in, 1 out]
    n198 = Scan Value(string=w406, format string="%f") -> (value=→"H2O":dbl)  [unwired: 1 in, 1 out]
    n199 = Scan Value(string=w411, format string="%f") -> (value=→"CO2":dbl)  [unwired: 1 in, 1 out]
    n200 = Scan Value(string=w414, format string="%f") -> (value=→"CH4":dbl)  [unwired: 1 in, 1 out]
    n201 = Scan Value(string=w544, format string="%f") -> (value=→"Std\nContent (barG)":dbl)  [unwired: 1 in, 1 out]
    n202 = Scan Value(string=w504, format string="%d", default (0 dbl)=u32 0) -> (value=w558:u32)  [unwired: 1 out]
    n203 = Scan Value(string=w543, format string="%f") -> (value=→"N2\nContent (barG)":dbl)  [unwired: 1 in, 1 out]
    n204 = Scan Value(string=w545, format string="%f") -> (value=→"CO2\nContent (barG)":dbl)  [unwired: 1 in, 1 out]
    n205 = Scan Value(string=w551, format string="%f") -> (value=→"CO2 Pressure\nDelivery (PSIA)":dbl)  [unwired: 1 in, 1 out]
    n206 = To Time Stamp(1:w421) -> (0:w428:timestamp)
    n207 = Scan Value(string=w473, format string="%f") -> (value=→"TEi49C Concentration":dbl)  [unwired: 1 in, 1 out]
    n208 = Scan Value(string=w472, format string="%f") -> (value=→"TEI49C Sample Flow A":dbl)  [unwired: 1 in, 1 out]
    n209 = Scan Value(string=w492, format string="%f") -> (value=→"Lamp Flow Controller":dbl)  [unwired: 1 in, 1 out]
    n210 = Scan Value(string=w359, format string="%f") -> (value=→"Raw Signal":dbl)  [unwired: 1 in, 1 out]
    n211 = Scan Value(string=w378, format string="%f") -> (value=→"CO Concentration":dbl)  [unwired: 1 in, 1 out]
    n212 = Scan Value(string=w471, format string="%f") -> (value=→"TEI49C Sample Flow B":dbl)  [unwired: 1 in, 1 out]
    n213 = Scan Value(string=w489, format string="%f") -> (value=→"Monochromater Flow":dbl)  [unwired: 1 in, 1 out]
    n214 = Scan Value(string=w488, format string="%f") -> (value=→"Fluorsecence Cell Pressure":dbl)  [unwired: 1 in, 1 out]
    n215 = Not Equal To 0?(x=w558) -> (x != 0?=→"CO CAL Status":bool)
    n216 = call "ping.vi"("Host IP Address"="192.168.101.17") -> ("connected?"=w427:bool)  [unwired: 14 in]
    n217 = Scan Value(string=w448, format string="%f") -> (value=w439:dbl)  [unwired: 1 in, 1 out]
    n218 = Scan Value(string=w447, format string="%f") -> (value=w431:dbl)  [unwired: 1 in, 1 out]
    n219 = Not Equal?(x=w438, y=w439) -> (x != y?=w444:bool)
    n220 = Not Equal?(x=w429, y=w431) -> (x != y?=w436:bool)
    n221 = case shown="True" w444 {
      tunnel: w445 -> [w619 w628]
      tunnel: w443 -> [w620 w627]
      tunnel: [w620 w626] -> w442
      tunnel: w428 -> [_ w622]
      tunnel: w439 -> [_ w623]
      tunnel: [w619 w625] -> w441
      tunnel: [w618 w624] -> w440
      tunnel: w439 -> [_ w624]
      tunnel: w438 -> [w618 _]
      frame False {
      }
      frame True {
        n222 = Bundle(w622, w623) -> (w621:cluster{timestamp, dbl})  [unwired: 1 in]
        n223 = Replace Array Subset(array=w628, new element=w621, index=w627) -> (w625:cluster{"time stamp":timestamp, "Y":dbl}[])
        n224 = Increment(x=w627) -> (x+1=w626:i32)
      }
    }
    "CO Sensitivity" <- w441
    n225 = case shown="True" w436 {
      tunnel: w435 -> [w608 w617]
      tunnel: w434 -> [w609 w616]
      tunnel: [w609 w615] -> w432
      tunnel: w428 -> [_ w614]
      tunnel: w431 -> [_ w613]
      tunnel: [w608 w612] -> w433
      tunnel: [w607 w611] -> w430
      tunnel: w431 -> [_ w611]
      tunnel: w429 -> [w607 _]
      frame False {
      }
      frame True {
        n226 = Bundle(w614, w613) -> (w610:cluster{timestamp, dbl})  [unwired: 1 in]
        n227 = Replace Array Subset(array=w617, new element=w610, index=w616) -> (w612:cluster{"time stamp":timestamp, "Y":dbl}[])
        n228 = Increment(x=w616) -> (x+1=w615:i32)
      }
    }
    "CO Zero" <- w433
    n229 = case shown="False" w427 {
      tunnel: w426 -> [_ w606]
      tunnel: [FALSE w603] -> w425
      frame False {
      }
      frame True {
        n230 = Select(t=FALSE, s=w606, f=TRUE) -> (s? t:f=w603:bool)
      }
    }
    "Network to cRIO live status" <- w425
    n231 = Wait (ms)(milliseconds to wait=u32 1000) -> ()  [unwired: 1 out]
  }
  n232 = while {
    stop <- FALSE stop-if-true
    # "Preflight Sub VI Descriptions"
    n233 = case shown="True" "Postflight Procedures" {
      frame False {
      }
      frame True {
        n234 = call "PostFlight Procedures.vi"() -> ()  [unwired: 12 in]
      }
    }
    n235 = case shown="True" "Prepare Gases" {
      frame False {
      }
      frame True {
        n236 = call "CO Gas Preparation.vi"() -> ()  [unwired: 12 in]
      }
    }
    n237 = Wait (ms)(milliseconds to wait=u32 500) -> ()  [unwired: 1 out]
  }
  n238 = Obtain Queue(name (unnamed)="FGGA_Command", element data type=w55) -> (queue out=w2:refnum<queue>, error out=w1:errorcluster)  [unwired: 3 in, 1 out]
  n239 = while {
    shift-right: [w636] -> _
    shift-left: u8 1 -> [w637]
    tunnel: w2 -> [w634]
    tunnel: w1 -> [w633]
    stop <- FALSE stop-if-true
    # "FGGA pump synchronise to WoW Wait on Wheel Flag"
    n240 = Wait (ms)(milliseconds to wait=u32 1000) -> ()  [unwired: 1 out]
    n241 = case shown="True" "FGGA pump\nsync to WoW" {
      tunnel: [w640 w645] -> w636
      tunnel: w637 -> [w640 w644]
      tunnel: w634 -> [_ w643]
      tunnel: w633 -> [_ w642]
      frame False {
      }
      frame True {
        n242 = local read "WoW Flag"() -> (w641:string)
        n243 = Scan Value(string=w641, format string="%d", default (0 dbl)=u8 0) -> (value=w645:u8)  [unwired: 1 out]
        n244 = Not Equal?(x=w645, y=w644) -> (x != y?=w648:bool)
        n245 = case shown="True" w648 {
          tunnel: w645 -> [_ w651]
          tunnel: w643 -> [_ w650]
          tunnel: w642 -> [_ w649]
          frame False {
          }
          frame True {
            n246 = Equal?(x=w651, y=u8 0) -> (x = y?=w656:bool)
            n247 = case shown="True" w656 {
              selector: w656 -> [w658 w659]
              tunnel: [w658 w659] -> w652
              frame False {
              }
              frame True {
              }
            }
            n248 = local write "Manual FGGA Pump"(w652) -> ()
            n249 = Bundle(cluster=T4 {"Message"="", "Message Data"=variant} ("Message Cluster"), "Message"="FGGA_pump", "Message Data"=w652) -> (w653:T4)
            n250 = Enqueue Element(queue=w650, element=w653, error in (no error)=w649) -> ()  [unwired: 1 in, 3 out]
          }
        }
      }
    }
  }
  n251 = while {
    tunnel: w2 -> [w661]
    tunnel: w1 -> [w660]
    tunnel: [w663] -> _
    tunnel: w13 -> [w662]
    stop <- FALSE stop-if-true
    # "FGGA UI Event Handler Loop"
    n252 = event shown="[12] \"Flush Target Tank\": Value Change" {
      selector: _ -> [_ _ _ _ _ _ _ _ _ _ _ _ _ _ _ _ _]
      dyn-events: _ -> [_ _ _ _ _ _ _ _ _ _ _ _ _ _ _ _ _]
      timeout: _ -> [_ _ _ _ _ _ _ _ _ _ _ _ _ _ _ _ _]
      tunnel: w661 -> [w671 w675 w682 w689 w696 w703 w710 w717 w736 w845 w1018 w1085 w1152 w1209 w1296 w1364 w1371]
      tunnel: w660 -> [w670 w674 w681 w688 w695 w702 w709 w716 w735 w844 w1017 w1084 w1151 w1208 w1295 w1363 w1370]
      tunnel: [w665 w673 w680 w687 w694 w701 w708 w715 w722 w808 w1010 w1077 w1144 w1195 w1282 w1362 w1369] -> w663
      tunnel: w662 -> [_ _ _ _ _ _ _ _ _ w832 _ _ _ _ _ _ _]
      event "eV1": Value Change {
        n253 = event-data() -> ("NewVal"=w668:bool)  [unwired: 1 in]
        n254 = Bundle(cluster=T4 {"Message"="", "Message Data"=variant} ("Message Cluster"), "Message"="V1", "Message Data"=w668) -> (w666:T4)
        n255 = Enqueue Element(queue=w671, element=w666, error in (no error)=w670) -> (error out=w665:errorcluster)  [unwired: 1 in, 2 out]
      }
      event "eV2": Value Change {
        n256 = event-data() -> ("NewVal"=w672:bool)  [unwired: 1 in]
        n257 = Bundle(cluster=T4 {"Message"="", "Message Data"=variant} ("Message Cluster"), "Message"="V2", "Message Data"=w672) -> (w676:T4)
        n258 = Enqueue Element(queue=w675, element=w676, error in (no error)=w674) -> (error out=w673:errorcluster)  [unwired: 1 in, 2 out]
      }
      event "eV3": Value Change {
        n259 = event-data() -> ("NewVal"=w679:bool)  [unwired: 1 in]
        n260 = Bundle(cluster=T4 {"Message"="", "Message Data"=variant} ("Message Cluster"), "Message"="V3", "Message Data"=w679) -> (w683:T4)
        n261 = Enqueue Element(queue=w682, element=w683, error in (no error)=w681) -> (error out=w680:errorcluster)  [unwired: 1 in, 2 out]
      }
      event "eV4": Value Change {
        n262 = event-data() -> ("NewVal"=w686:bool)  [unwired: 1 in]
        n263 = Bundle(cluster=T4 {"Message"="", "Message Data"=variant} ("Message Cluster"), "Message"="V4", "Message Data"=w686) -> (w690:T4)
        n264 = Enqueue Element(queue=w689, element=w690, error in (no error)=w688) -> (error out=w687:errorcluster)  [unwired: 1 in, 2 out]
      }
      event "Manual FGGA Pump": Value Change {
        n265 = event-data() -> ("NewVal"=w693:bool)  [unwired: 1 in]
        n266 = Bundle(cluster=T4 {"Message"="", "Message Data"=variant} ("Message Cluster"), "Message"="FGGA_pump", "Message Data"=w693) -> (w697:T4)
        n267 = Enqueue Element(queue=w696, element=w697, error in (no error)=w695) -> (error out=w694:errorcluster)  [unwired: 1 in, 2 out]
      }
      event "Confirm Flight Number": Value Change {
        n268 = event-data() -> ()  [unwired: 1 in, 6 out]
        n269 = local read "Flight Number"() -> (w700:string)
        n270 = Bundle(cluster=T4 {"Message"="", "Message Data"=variant} ("Message Cluster"), "Message"="Flight Number", "Message Data"=w700) -> (w704:T4)
        n271 = Enqueue Element(queue=w703, element=w704, error in (no error)=w702) -> (error out=w701:errorcluster)  [unwired: 1 in, 2 out]
      }
      event "FGGA Restart": Value Change {
        n272 = event-data() -> ("NewVal"=w707:bool)  [unwired: 1 in]
        n273 = Bundle(cluster=T4 {"Message"="", "Message Data"=variant} ("Message Cluster"), "Message"="FGGA_restart", "Message Data"=w707) -> (w711:T4)
        n274 = Enqueue Element(queue=w710, element=w711, error in (no error)=w709) -> (error out=w708:errorcluster)  [unwired: 1 in, 2 out]
      }
      event "cRIO File IO Stop\n(USB Flash Drive Unmount)": Value Change {
        n275 = event-data() -> ("NewVal"=w714:bool)  [unwired: 1 in]
        n276 = Bundle(cluster=T4 {"Message"="", "Message Data"=variant} ("Message Cluster"), "Message"="Stop File Write", "Message Data"=w714) -> (w718:T4)
        n277 = Enqueue Element(queue=w717, element=w718, error in (no error)=w716) -> (error out=w715:errorcluster)  [unwired: 1 in, 2 out]
      }
      event "High Cal": Value Change {
        n278 = event-data() -> ()  [unwired: 1 in, 1 out]
        n279 = flat-sequence {
          tunnel: w736 -> [w741]
          tunnel: w735 -> [w740]
          tunnel: [w739] -> w734
          tunnel: [w738] -> w733
          tunnel: w734 -> [w757]
          tunnel: w733 -> [w756]
          tunnel: [w754] -> w731
          tunnel: [w753] -> w729
          tunnel: [w762] -> w732
          tunnel: w731 -> [w762]
          tunnel: [w761] -> w730
          tunnel: w729 -> [w761]
          tunnel: w732 -> [w772]
          tunnel: w730 -> [w771]
          tunnel: [w769] -> w727
          tunnel: [w768] -> w725
          tunnel: [w778] -> w728
          tunnel: w727 -> [w778]
          tunnel: [w777] -> w726
          tunnel: w725 -> [w777]
          tunnel: w728 -> [w788]
          tunnel: w726 -> [w787]
          tunnel: [w785] -> w724
          tunnel: [w784] -> w723
          tunnel: w724 -> [w802]
          tunnel: w723 -> [w801]
          tunnel: [w799] -> w721
          tunnel: [w807] -> w722
          tunnel: w721 -> [w807]
          frame #0 {
            w737 = TRUE
            n280 = Cluster To Array(cluster=T11 {"Message"="V2", "Message 2"="V3", "Message 3"="V4"}) -> (array=w742:string[])
            n281 = for {
              tunnel: w742 -> [w749] mode=indexing
              tunnel: w741 -> [w748]
              tunnel: w740 -> [w747]
              tunnel: [w746] -> w739
              tunnel: [w745] -> w738
              tunnel: w737 -> [w744]
              n282 = Bundle(cluster=T4 {"Message"="", "Message Data"=variant} ("Message Cluster"), "Message"=w749, "Message Data"=w744) -> (w751:T4)
              n283 = Enqueue Element(queue=w748, element=w751, error in (no error)=w747) -> (queue out=w746:refnum<queue>, error out=w745:errorcluster)  [unwired: 1 in, 1 out]
            }
            n284 = local write "eV2"(w737) -> ()
            n285 = local write "eV4"(w737) -> ()
            n286 = local write "eV3"(w737) -> ()
          }
          frame #1 {
            n287 = local read "MFC_1 User Set Value"() -> (w752:dbl)
            n288 = local write "MFC_1\nSLPM Value"(w752) -> ()
            n289 = Bundle(cluster=T4 {"Message"="", "Message Data"=variant} ("Message Cluster"), "Message"="MFC_1", "Message Data"=w752) -> (w755:T4)
            n290 = Enqueue Element(queue=w757, element=w755, error in (no error)=w756) -> (queue out=w754:refnum<queue>, error out=w753:errorcluster)  [unwired: 1 in, 1 out]
          }
          frame #2 {
            n291 = for {
              N: 45 -> [w766]
              i -> [w765]
              n292 = Subtract(x=w766, y=w765) -> (x-y=w764:i32)
              n293 = Decrement(x=w764) -> (x-1=→"High Cal\nFlush Time Remain (sec)":i32)
              n294 = Wait (ms)(milliseconds to wait=u32 1000) -> ()  [unwired: 1 out]
            }
          }
          frame #3 {
            w770 = TRUE
            n295 = Bundle(cluster=T4 {"Message"="", "Message Data"=variant} ("Message Cluster"), "Message"="V1", "Message Data"=w770) -> (w773:T4)
            n296 = local write "eV1"(w770) -> ()
            n297 = Enqueue Element(queue=w772, element=w773, error in (no error)=w771) -> (queue out=w769:refnum<queue>, error out=w768:errorcluster)  [unwired: 1 in, 1 out]
          }
          frame #4 {
            n298 = for {
              N: 60 -> [w782]
              i -> [w781]
              n299 = Subtract(x=w782, y=w781) -> (x-y=w780:i32)
              n300 = Decrement(x=w780) -> (x-1=→"High Cal\nCal Time Remain (sec)":i32)
              n301 = Wait (ms)(milliseconds to wait=u32 1000) -> ()  [unwired: 1 out]
            }
          }
          frame #5 {
            w786 = FALSE
            n302 = Cluster To Array(cluster=T12 {"Message"="V2", "Message 2"="V3", "Message 3"="V4", "Message 4"="V1"}) -> (array=w789:string[])
            n303 = for {
              tunnel: w789 -> [w796] mode=indexing
              tunnel: [w795] -> w785
              tunnel: [w794] -> w784
              tunnel: w786 -> [w793]
              tunnel: w788 -> [w792]
              tunnel: w787 -> [w791]
              n304 = Bundle(cluster=T4 {"Message"="", "Message Data"=variant} ("Message Cluster"), "Message"=w796, "Message Data"=w793) -> (w798:T4)
              n305 = Enqueue Element(queue=w792, element=w798, error in (no error)=w791) -> (queue out=w795:refnum<queue>, error out=w794:errorcluster)  [unwired: 1 in, 1 out]
            }
            n306 = local write "eV2"(w786) -> ()
            n307 = local write "eV4"(w786) -> ()
            n308 = local write "eV3"(w786) -> ()
            n309 = local write "eV1"(w786) -> ()
          }
          frame #6 {
            w800 = 0.0 ("MFC_1\nSLPM Value")
            n310 = local write "MFC_1\nSLPM Value"(w800) -> ()
            n311 = Bundle(cluster=T4 {"Message"="", "Message Data"=variant} ("Message Cluster"), "Message"="MFC_1", "Message Data"=w800) -> (w804:T4)
            n312 = Enqueue Element(queue=w802, element=w804, error in (no error)=w801) -> (error out=w799:errorcluster)  [unwired: 1 in, 2 out]
          }
          frame #7 {
            n313 = local write "High Cal"(FALSE ("High Cal")) -> ()
          }
        }
      }
      event "Span Cal - \nHigh Cal, CO Cal, Low Cal": Value Change {
        n314 = event-data() -> ()  [unwired: 1 in, 1 out]
        n315 = flat-sequence {
          tunnel: w845 -> [w851]
          tunnel: w844 -> [w850]
          tunnel: [w849] -> w843
          tunnel: [w848] -> w842
          tunnel: w843 -> [w867]
          tunnel: w842 -> [w866]
          tunnel: [w864] -> w840
          tunnel: [w863] -> w838
          tunnel: [w872] -> w841
          tunnel: w840 -> [w872]
          tunnel: [w871] -> w839
          tunnel: w838 -> [w871]
          tunnel: w841 -> [w878]
          tunnel: w839 -> [w879]
          tunnel: [w879] -> w814
          tunnel: w832 -> [w880]
          tunnel: [w880] -> w812
          tunnel: [w878] -> w810
          tunnel: w814 -> [w888]
          tunnel: [w888] -> w813
          tunnel: w812 -> [w887]
          tunnel: [w887] -> w811
          tunnel: w810 -> [w885]
          tunnel: [w885] -> w809
          tunnel: [w889] -> w831
          tunnel: w813 -> [w892]
          tunnel: [w891] -> w830
          tunnel: w811 -> [w901]
          tunnel: w809 -> [w890]
          tunnel: [w904] -> w837
          tunnel: w831 -> [w904]
          tunnel: [w903] -> w836
          tunnel: w830 -> [w903]
          tunnel: w837 -> [w914]
          tunnel: w836 -> [w913]
          tunnel: [w911] -> w835
          tunnel: [w910] -> w834
          tunnel: w835 -> [w929]
          tunnel: w834 -> [w928]
          tunnel: [w926] -> w833
          tunnel: [w925] -> w827
          tunnel: w833 -> [w935]
          tunnel: [w935] -> w829
          tunnel: [w933] -> w828
          tunnel: w827 -> [w933]
          tunnel: w829 -> [w940]
          tunnel: w828 -> [w942]
          tunnel: [w939] -> w826
          tunnel: [w936] -> w825
          tunnel: w826 -> [w956]
          tunnel: w825 -> [w954]
          tunnel: [w953] -> w824
          tunnel: [w952] -> w821
          tunnel: w824 -> [w961]
          tunnel: [w961] -> w823
          tunnel: [w960] -> w822
          tunnel: w821 -> [w960]
          tunnel: w823 -> [w973]
          tunnel: w822 -> [w971]
          tunnel: [w969] -> w819
          tunnel: [w968] -> w817
          tunnel: [w977] -> w820
          tunnel: w819 -> [w977]
          tunnel: [w976] -> w818
          tunnel: w817 -> [w976]
          tunnel: w820 -> [w988]
          tunnel: w818 -> [w987]
          tunnel: [w985] -> w816
          tunnel: [w984] -> w815
          tunnel: w816 -> [w1003]
          tunnel: w815 -> [w1002]
          tunnel: [w999] -> w808
          frame #0 {
            w847 = TRUE
            n316 = Cluster To Array(cluster=T11 {"Message"="V2", "Message 2"="V3", "Message 3"="V4"}) -> (array=w852:string[])
            n317 = for {
              tunnel: w852 -> [w859] mode=indexing
              tunnel: w851 -> [w858]
              tunnel: w850 -> [w857]
              tunnel: [w856] -> w849
              tunnel: [w855] -> w848
              tunnel: w847 -> [w854]
              n318 = Bundle(cluster=T4 {"Message"="", "Message Data"=variant} ("Message Cluster"), "Message"=w859, "Message Data"=w854) -> (w861:T4)
              n319 = Enqueue Element(queue=w858, element=w861, error in (no error)=w857) -> (queue out=w856:refnum<queue>, error out=w855:errorcluster)  [unwired: 1 in, 1 out]
            }
            n320 = local write "High Cal"(TRUE ("High Cal")) -> ()
            n321 = local write "eV2"(w847) -> ()
            n322 = local write "eV4"(w847) -> ()
            n323 = local write "eV3"(w847) -> ()
          }
          frame #1 {
            n324 = local read "MFC_1 User Set Value"() -> (w862:dbl)
            n325 = local write "MFC_1\nSLPM Value"(w862) -> ()
            n326 = Bundle(cluster=T4 {"Message"="", "Message Data"=variant} ("Message Cluster"), "Message"="MFC_1", "Message Data"=w862) -> (w865:T4)
            n327 = Enqueue Element(queue=w867, element=w865, error in (no error)=w866) -> (queue out=w864:refnum<queue>, error out=w863:errorcluster)  [unwired: 1 in, 1 out]
          }
          frame #2 {
            n328 = for {
              N: 45 -> [w876]
              i -> [w875]
              n329 = Subtract(x=w876, y=w875) -> (x-y=w874:i32)
              n330 = Decrement(x=w874) -> (x-1=w873:i32)
              n331 = local write "High Cal\nFlush Time Remain (sec)"(w873) -> ()
              n332 = Wait (ms)(milliseconds to wait=u32 1000) -> ()  [unwired: 1 out]
            }
          }
          frame #3 {
            n333 = Bundle(cluster=T4 {"Message"="", "Message Data"=variant} ("Message Cluster"), "Message"="CO CAL", "Message Data"=TRUE) -> (w882:T4)
            n334 = Enqueue Element(queue=w880, element=w882) -> ()  [unwired: 2 in, 3 out]
          }
          frame #4 {
            # "To Ensure\nCO CAL\nis certain"
            n335 = Wait (ms)(milliseconds to wait=u32 1000) -> ()  [unwired: 1 out]
          }
          frame #5 {
            w896 = TRUE
            n336 = Bundle(cluster=T4 {"Message"="", "Message Data"=variant} ("Message Cluster"), "Message"="CO CAL", "Message Data"=FALSE) -> (w897:T4)
            n337 = Bundle(cluster=T4 {"Message"="", "Message Data"=variant} ("Message Cluster"), "Message"="V1", "Message Data"=w896) -> (w895:T4)
            n338 = local write "eV1"(w896) -> ()
            n339 = Enqueue Element(queue=w901, element=w897) -> ()  [unwired: 2 in, 3 out]
            n340 = Enqueue Element(queue=w890, element=w895, error in (no error)=w892) -> (queue out=w889:refnum<queue>, error out=w891:errorcluster)  [unwired: 1 in, 1 out]
          }
          frame #6 {
            n341 = for {
              N: 60 -> [w908]
              i -> [w907]
              n342 = Subtract(x=w908, y=w907) -> (x-y=w906:i32)
              n343 = Decrement(x=w906) -> (x-1=w905:i32)
              n344 = local write "High Cal\nCal Time Remain (sec)"(w905) -> ()
              n345 = Wait (ms)(milliseconds to wait=u32 1000) -> ()  [unwired: 1 out]
            }
          }
          frame #7 {
            w912 = FALSE
            n346 = Cluster To Array(cluster=T12 {"Message"="V2", "Message 2"="V3", "Message 3"="V4", "Message 4"="V1"}) -> (array=w915:string[])
            n347 = for {
              tunnel: w915 -> [w922] mode=indexing
              tunnel: [w921] -> w911
              tunnel: [w920] -> w910
              tunnel: w912 -> [w919]
              tunnel: w914 -> [w918]
              tunnel: w913 -> [w917]
              n348 = Bundle(cluster=T4 {"Message"="", "Message Data"=variant} ("Message Cluster"), "Message"=w922, "Message Data"=w919) -> (w924:T4)
              n349 = Enqueue Element(queue=w918, element=w924, error in (no error)=w917) -> (queue out=w921:refnum<queue>, error out=w920:errorcluster)  [unwired: 1 in, 1 out]
            }
            n350 = local write "eV2"(w912) -> ()
            n351 = local write "eV4"(w912) -> ()
            n352 = local write "eV3"(w912) -> ()
            n353 = local write "eV1"(w912) -> ()
          }
          frame #8 {
            w927 = 0.0 ("MFC_1\nSLPM Value")
            n354 = local write "MFC_1\nSLPM Value"(w927) -> ()
            n355 = Bundle(cluster=T4 {"Message"="", "Message Data"=variant} ("Message Cluster"), "Message"="MFC_1", "Message Data"=w927) -> (w931:T4)
            n356 = Enqueue Element(queue=w929, element=w931, error in (no error)=w928) -> (queue out=w925:refnum<queue>, error out=w926:errorcluster)  [unwired: 1 in, 1 out]
          }
          frame #9 {
            n357 = local write "High Cal"(FALSE ("High Cal")) -> ()
          }
          frame #10 {
            w937 = TRUE
            n358 = Cluster To Array(cluster=cluster{"Message":string, "Message 3":string} {"Message"="V2", "Message 3"="V4"}) -> (array=w943:string[])
            n359 = for {
              tunnel: w943 -> [w949] mode=indexing
              tunnel: w942 -> [w948]
              tunnel: [w947] -> w936
              tunnel: [w946] -> w939
              tunnel: w937 -> [w945]
              tunnel: w940 -> [w944]
              n360 = Bundle(cluster=T4 {"Message"="", "Message Data"=variant} ("Message Cluster"), "Message"=w949, "Message Data"=w945) -> (w951:T4)
              n361 = Enqueue Element(queue=w948, element=w951, error in (no error)=w944) -> (queue out=w947:refnum<queue>, error out=w946:errorcluster)  [unwired: 1 in, 1 out]
            }
            n362 = local write "eV4"(w937) -> ()
            n363 = local write "eV2"(w937) -> ()
            n364 = local write "Low Cal"(TRUE ("Low Cal")) -> ()
          }
          frame #11 {
            n365 = local read "MFC_1 User Set Value"() -> (w957:dbl)
            n366 = local write "MFC_1\nSLPM Value"(w957) -> ()
            n367 = Bundle(cluster=T4 {"Message"="", "Message Data"=variant} ("Message Cluster"), "Message"="MFC_1", "Message Data"=w957) -> (w958:T4)
            n368 = Enqueue Element(queue=w954, element=w958, error in (no error)=w956) -> (queue out=w953:refnum<queue>, error out=w952:errorcluster)  [unwired: 1 in, 1 out]
          }
          frame #12 {
            n369 = for {
              N: 45 -> [w966]
              i -> [w965]
              n370 = Subtract(x=w966, y=w965) -> (x-y=w964:i32)
              n371 = Decrement(x=w964) -> (x-1=w963:i32)
              n372 = local write "Low Cal\nFlush Time Remain (sec)"(w963) -> ()
              n373 = Wait (ms)(milliseconds to wait=u32 1000) -> ()  [unwired: 1 out]
            }
          }
          frame #13 {
            w970 = TRUE
            n374 = local write "eV1"(w970) -> ()
            n375 = Bundle(cluster=T4 {"Message"="", "Message Data"=variant} ("Message Cluster"), "Message"="V1", "Message Data"=w970) -> (w974:T4)
            n376 = Enqueue Element(queue=w973, element=w974, error in (no error)=w971) -> (queue out=w969:refnum<queue>, error out=w968:errorcluster)  [unwired: 1 in, 1 out]
          }
          frame #14 {
            n377 = for {
              N: 60 -> [w982]
              i -> [w981]
              n378 = Subtract(x=w982, y=w981) -> (x-y=w980:i32)
              n379 = Decrement(x=w980) -> (x-1=w979:i32)
              n380 = local write "Low Cal\nCal Time Remain (sec)"(w979) -> ()
              n381 = Wait (ms)(milliseconds to wait=u32 1000) -> ()  [unwired: 1 out]
            }
          }
          frame #15 {
            w986 = FALSE
            n382 = Cluster To Array(cluster=T13 {"Message"="V2", "Message 3"="V4", "Message 4"="V1"}) -> (array=w989:string[])
            n383 = local write "eV1"(w986) -> ()
            n384 = local write "eV2"(w986) -> ()
            n385 = local write "eV4"(w986) -> ()
            n386 = for {
              tunnel: w989 -> [w996] mode=indexing
              tunnel: [w995] -> w985
              tunnel: [w994] -> w984
              tunnel: w986 -> [w993]
              tunnel: w988 -> [w992]
              tunnel: w987 -> [w991]
              n387 = Bundle(cluster=T4 {"Message"="", "Message Data"=variant} ("Message Cluster"), "Message"=w996, "Message Data"=w993) -> (w998:T4)
              n388 = Enqueue Element(queue=w992, element=w998, error in (no error)=w991) -> (queue out=w995:refnum<queue>, error out=w994:errorcluster)  [unwired: 1 in, 1 out]
            }
          }
          frame #16 {
            w1000 = FALSE
            w1001 = 0.0 ("MFC_1\nSLPM Value")
            n389 = local write "Span Cal - \nHigh Cal, CO Cal, Low Cal"(w1000) -> ()
            n390 = local write "MFC_1\nSLPM Value"(w1001) -> ()
            n391 = local write "Low Cal"(w1000) -> ()
            n392 = Bundle(cluster=T4 {"Message"="", "Message Data"=variant} ("Message Cluster"), "Message"="MFC_1", "Message Data"=w1001) -> (w1005:T4)
            n393 = Enqueue Element(queue=w1003, element=w1005, error in (no error)=w1002) -> (error out=w999:errorcluster)  [unwired: 1 in, 2 out]
          }
        }
      }
      event "Flush High Tank": Value Change {
        n394 = event-data() -> ()  [unwired: 1 in, 1 out]
        n395 = flat-sequence {
          tunnel: w1018 -> [w1023]
          tunnel: w1017 -> [w1022]
          tunnel: [w1021] -> w1016
          tunnel: [w1020] -> w1015
          tunnel: w1016 -> [w1039]
          tunnel: w1015 -> [w1038]
          tunnel: [w1036] -> w1014
          tunnel: [w1035] -> w1013
          tunnel: w1014 -> [w1042]
          tunnel: w1013 -> [w1043]
          tunnel: [w1043] -> w1008
          tunnel: [w1042] -> w1007
          tunnel: [w1053] -> w1012
          tunnel: [w1052] -> w1011
          tunnel: w1008 -> [w1051]
          tunnel: w1007 -> [w1050]
          tunnel: w1012 -> [w1068]
          tunnel: w1011 -> [w1067]
          tunnel: [w1065] -> w1009
          tunnel: [w1073] -> w1010
          tunnel: w1009 -> [w1073]
          frame #0 {
            w1019 = TRUE
            n396 = Cluster To Array(cluster=T11 {"Message"="V2", "Message 2"="V3", "Message 3"="V4"}) -> (array=w1024:string[])
            n397 = for {
              tunnel: w1024 -> [w1031] mode=indexing
              tunnel: w1023 -> [w1030]
              tunnel: w1022 -> [w1029]
              tunnel: [w1028] -> w1021
              tunnel: [w1027] -> w1020
              tunnel: w1019 -> [w1026]
              n398 = Bundle(cluster=T4 {"Message"="", "Message Data"=variant} ("Message Cluster"), "Message"=w1031, "Message Data"=w1026) -> (w1033:T4)
              n399 = Enqueue Element(queue=w1030, element=w1033, error in (no error)=w1029) -> (queue out=w1028:refnum<queue>, error out=w1027:errorcluster)  [unwired: 1 in, 1 out]
            }
            n400 = local write "eV2"(w1019) -> ()
            n401 = local write "eV4"(w1019) -> ()
            n402 = local write "eV3"(w1019) -> ()
          }
          frame #1 {
            n403 = local read "MFC_1 User Set Value"() -> (w1034:dbl)
            n404 = local write "MFC_1\nSLPM Value"(w1034) -> ()
            n405 = Bundle(cluster=T4 {"Message"="", "Message Data"=variant} ("Message Cluster"), "Message"="MFC_1", "Message Data"=w1034) -> (w1037:T4)
            n406 = Enqueue Element(queue=w1039, element=w1037, error in (no error)=w1038) -> (queue out=w1036:refnum<queue>, error out=w1035:errorcluster)  [unwired: 1 in, 1 out]
          }
          frame #2 {
            n407 = for {
              N: 15 -> [w1048]
              i -> [w1047]
              n408 = Subtract(x=w1048, y=w1047) -> (x-y=w1046:i32)
              n409 = Decrement(x=w1046) -> (x-1=→"Flush High Tank\nTime Remain (sec)":i32)
              n410 = Wait (ms)(milliseconds to wait=u32 1000) -> ()  [unwired: 1 out]
            }
          }
          frame #3 {
            w1054 = FALSE
            n411 = Cluster To Array(cluster=T11 {"Message"="V2", "Message 2"="V3", "Message 3"="V4"}) -> (array=w1055:string[])
            n412 = for {
              tunnel: w1055 -> [w1062] mode=indexing
              tunnel: [w1061] -> w1053
              tunnel: [w1060] -> w1052
              tunnel: w1054 -> [w1059]
              tunnel: w1050 -> [w1058]
              tunnel: w1051 -> [w1057]
              n413 = Bundle(cluster=T4 {"Message"="", "Message Data"=variant} ("Message Cluster"), "Message"=w1062, "Message Data"=w1059) -> (w1064:T4)
              n414 = Enqueue Element(queue=w1058, element=w1064, error in (no error)=w1057) -> (queue out=w1061:refnum<queue>, error out=w1060:errorcluster)  [unwired: 1 in, 1 out]
            }
            n415 = local write "eV2"(w1054) -> ()
            n416 = local write "eV4"(w1054) -> ()
            n417 = local write "eV3"(w1054) -> ()
          }
          frame #4 {
            w1066 = 0.0 ("MFC_1\nSLPM Value")
            n418 = local write "MFC_1\nSLPM Value"(w1066) -> ()
            n419 = Bundle(cluster=T4 {"Message"="", "Message Data"=variant} ("Message Cluster"), "Message"="MFC_1", "Message Data"=w1066) -> (w1070:T4)
            n420 = Enqueue Element(queue=w1068, element=w1070, error in (no error)=w1067) -> (error out=w1065:errorcluster)  [unwired: 1 in, 2 out]
          }
          frame #5 {
            n421 = local write "Flush High Tank"(FALSE ("High Cal")) -> ()
          }
        }
      }
      event "Flush Low Tank": Value Change {
        n422 = event-data() -> ()  [unwired: 1 in, 1 out]
        n423 = flat-sequence {
          tunnel: w1085 -> [w1090]
          tunnel: w1084 -> [w1089]
          tunnel: [w1088] -> w1083
          tunnel: [w1087] -> w1082
          tunnel: w1083 -> [w1106]
          tunnel: w1082 -> [w1105]
          tunnel: [w1103] -> w1081
          tunnel: [w1102] -> w1080
          tunnel: w1081 -> [w1109]
          tunnel: w1080 -> [w1110]
          tunnel: [w1110] -> w1075
          tunnel: [w1109] -> w1074
          tunnel: [w1120] -> w1079
          tunnel: [w1119] -> w1078
          tunnel: w1075 -> [w1118]
          tunnel: w1074 -> [w1117]
          tunnel: w1079 -> [w1135]
          tunnel: w1078 -> [w1134]
          tunnel: [w1132] -> w1076
          tunnel: [w1140] -> w1077
          tunnel: w1076 -> [w1140]
          frame #0 {
            w1086 = TRUE
            n424 = Cluster To Array(cluster=cluster{"Message":string, "Message 3":string} {"Message"="V2", "Message 3"="V4"}) -> (array=w1091:string[])
            n425 = for {
              tunnel: w1091 -> [w1098] mode=indexing
              tunnel: w1090 -> [w1097]
              tunnel: w1089 -> [w1096]
              tunnel: [w1095] -> w1088
              tunnel: [w1094] -> w1087
              tunnel: w1086 -> [w1093]
              n426 = Bundle(cluster=T4 {"Message"="", "Message Data"=variant} ("Message Cluster"), "Message"=w1098, "Message Data"=w1093) -> (w1100:T4)
              n427 = Enqueue Element(queue=w1097, element=w1100, error in (no error)=w1096) -> (queue out=w1095:refnum<queue>, error out=w1094:errorcluster)  [unwired: 1 in, 1 out]
            }
            n428 = local write "eV2"(w1086) -> ()
            n429 = local write "eV4"(w1086) -> ()
          }
          frame #1 {
            n430 = local read "MFC_1 User Set Value"() -> (w1101:dbl)
            n431 = local write "MFC_1\nSLPM Value"(w1101) -> ()
            n432 = Bundle(cluster=T4 {"Message"="", "Message Data"=variant} ("Message Cluster"), "Message"="MFC_1", "Message Data"=w1101) -> (w1104:T4)
            n433 = Enqueue Element(queue=w1106, element=w1104, error in (no error)=w1105) -> (queue out=w1103:refnum<queue>, error out=w1102:errorcluster)  [unwired: 1 in, 1 out]
          }
          frame #2 {
            n434 = for {
              N: 15 -> [w1115]
              i -> [w1114]
              n435 = Subtract(x=w1115, y=w1114) -> (x-y=w1113:i32)
              n436 = Decrement(x=w1113) -> (x-1=→"Flush Low Tank\nTime Remain (sec)":i32)
              n437 = Wait (ms)(milliseconds to wait=u32 1000) -> ()  [unwired: 1 out]
            }
          }
          frame #3 {
            w1121 = FALSE
            n438 = Cluster To Array(cluster=cluster{"Message":string, "Message 3":string} {"Message"="V2", "Message 3"="V4"}) -> (array=w1122:string[])
            n439 = for {
              tunnel: w1122 -> [w1129] mode=indexing
              tunnel: [w1128] -> w1120
              tunnel: [w1127] -> w1119
              tunnel: w1121 -> [w1126]
              tunnel: w1117 -> [w1125]
              tunnel: w1118 -> [w1124]
              n440 = Bundle(cluster=T4 {"Message"="", "Message Data"=variant} ("Message Cluster"), "Message"=w1129, "Message Data"=w1126) -> (w1131:T4)
              n441 = Enqueue Element(queue=w1125, element=w1131, error in (no error)=w1124) -> (queue out=w1128:refnum<queue>, error out=w1127:errorcluster)  [unwired: 1 in, 1 out]
            }
            n442 = local write "eV2"(w1121) -> ()
            n443 = local write "eV4"(w1121) -> ()
          }
          frame #4 {
            w1133 = 0.0 ("MFC_1\nSLPM Value")
            n444 = local write "MFC_1\nSLPM Value"(w1133) -> ()
            n445 = Bundle(cluster=T4 {"Message"="", "Message Data"=variant} ("Message Cluster"), "Message"="MFC_1", "Message Data"=w1133) -> (w1137:T4)
            n446 = Enqueue Element(queue=w1135, element=w1137, error in (no error)=w1134) -> (error out=w1132:errorcluster)  [unwired: 1 in, 2 out]
          }
          frame #5 {
            n447 = local write "Flush Low Tank"(FALSE ("High Cal")) -> ()
          }
        }
      }
      event "Flush Target Tank": Value Change {
        n448 = event-data() -> ()  [unwired: 1 in, 1 out]
        n449 = flat-sequence {
          tunnel: w1152 -> [w1160]
          tunnel: w1151 -> [w1159]
          tunnel: [w1158] -> w1150
          tunnel: [w1157] -> w1149
          tunnel: w1150 -> [w1166]
          tunnel: w1149 -> [w1165]
          tunnel: [w1163] -> w1148
          tunnel: [w1162] -> w1147
          tunnel: w1148 -> [w1169]
          tunnel: w1147 -> [w1170]
          tunnel: [w1170] -> w1142
          tunnel: [w1169] -> w1141
          tunnel: [w1183] -> w1146
          tunnel: [w1182] -> w1145
          tunnel: w1142 -> [w1181]
          tunnel: w1141 -> [w1180]
          tunnel: w1146 -> [w1188]
          tunnel: w1145 -> [w1187]
          tunnel: [w1185] -> w1143
          tunnel: [w1193] -> w1144
          tunnel: w1143 -> [w1193]
          frame #0 {
            w1156 = TRUE
            n450 = local write "eV4"(w1156) -> ()
            n451 = Bundle(cluster=T4 {"Message"="", "Message Data"=variant} ("Message Cluster"), "Message"="V4" ("Message 3"), "Message Data"=w1156) -> (w1155:T4)
            n452 = Enqueue Element(queue=w1160, element=w1155, error in (no error)=w1159) -> (queue out=w1158:refnum<queue>, error out=w1157:errorcluster)  [unwired: 1 in, 1 out]
          }
          frame #1 {
            n453 = local read "MFC_1 User Set Value"() -> (w1161:dbl)
            n454 = local write "MFC_1\nSLPM Value"(w1161) -> ()
            n455 = Bundle(cluster=T4 {"Message"="", "Message Data"=variant} ("Message Cluster"), "Message"="MFC_1", "Message Data"=w1161) -> (w1164:T4)
            n456 = Enqueue Element(queue=w1166, element=w1164, error in (no error)=w1165) -> (queue out=w1163:refnum<queue>, error out=w1162:errorcluster)  [unwired: 1 in, 1 out]
          }
          frame #2 {
            n457 = for {
              N: 15 -> [w1175]
              i -> [w1174]
              n458 = Subtract(x=w1175, y=w1174) -> (x-y=w1173:i32)
              n459 = Decrement(x=w1173) -> (x-1=→"Flush Target Tank\nTime Remain (sec)":i32)
              n460 = Wait (ms)(milliseconds to wait=u32 1000) -> ()  [unwired: 1 out]
            }
          }
          frame #3 {
            w1184 = FALSE
            n461 = Bundle(cluster=T4 {"Message"="", "Message Data"=variant} ("Message Cluster"), "Message"="V4" ("Message 3"), "Message Data"=w1184) -> (w1179:T4)
            n462 = local write "eV4"(w1184) -> ()
            n463 = Enqueue Element(queue=w1180, element=w1179, error in (no error)=w1181) -> (queue out=w1183:refnum<queue>, error out=w1182:errorcluster)  [unwired: 1 in, 1 out]
          }
          frame #4 {
            w1186 = 0.0 ("MFC_1\nSLPM Value")
            n464 = local write "MFC_1\nSLPM Value"(w1186) -> ()
            n465 = Bundle(cluster=T4 {"Message"="", "Message Data"=variant} ("Message Cluster"), "Message"="MFC_1", "Message Data"=w1186) -> (w1190:T4)
            n466 = Enqueue Element(queue=w1188, element=w1190, error in (no error)=w1187) -> (error out=w1185:errorcluster)  [unwired: 1 in, 2 out]
          }
          frame #5 {
            n467 = local write "Flush Target Tank"(FALSE ("High Cal")) -> ()
          }
        }
      }
      event "Low Cal": Value Change {
        n468 = event-data() -> ()  [unwired: 1 in, 1 out]
        n469 = flat-sequence {
          tunnel: w1209 -> [w1214]
          tunnel: w1208 -> [w1213]
          tunnel: [w1212] -> w1207
          tunnel: [w1211] -> w1206
          tunnel: w1207 -> [w1230]
          tunnel: w1206 -> [w1229]
          tunnel: [w1227] -> w1204
          tunnel: [w1226] -> w1202
          tunnel: [w1235] -> w1205
          tunnel: w1204 -> [w1235]
          tunnel: [w1234] -> w1203
          tunnel: w1202 -> [w1234]
          tunnel: w1205 -> [w1245]
          tunnel: w1203 -> [w1244]
          tunnel: [w1242] -> w1200
          tunnel: [w1241] -> w1198
          tunnel: [w1251] -> w1201
          tunnel: w1200 -> [w1251]
          tunnel: [w1250] -> w1199
          tunnel: w1198 -> [w1250]
          tunnel: w1201 -> [w1261]
          tunnel: w1199 -> [w1260]
          tunnel: [w1258] -> w1197
          tunnel: [w1257] -> w1196
          tunnel: w1197 -> [w1275]
          tunnel: w1196 -> [w1274]
          tunnel: [w1272] -> w1194
          tunnel: [w1280] -> w1195
          tunnel: w1194 -> [w1280]
          frame #0 {
            w1210 = TRUE
            n470 = Cluster To Array(cluster=cluster{"Message":string, "Message 3":string} {"Message"="V2", "Message 3"="V4"}) -> (array=w1215:string[])
            n471 = for {
              tunnel: w1215 -> [w1222] mode=indexing
              tunnel: w1214 -> [w1221]
              tunnel: w1213 -> [w1220]
              tunnel: [w1219] -> w1212
              tunnel: [w1218] -> w1211
              tunnel: w1210 -> [w1217]
              n472 = Bundle(cluster=T4 {"Message"="", "Message Data"=variant} ("Message Cluster"), "Message"=w1222, "Message Data"=w1217) -> (w1224:T4)
              n473 = Enqueue Element(queue=w1221, element=w1224, error in (no error)=w1220) -> (queue out=w1219:refnum<queue>, error out=w1218:errorcluster)  [unwired: 1 in, 1 out]
            }
            n474 = local write "eV2"(w1210) -> ()
            n475 = local write "eV4"(w1210) -> ()
          }
          frame #1 {
            n476 = local read "MFC_1 User Set Value"() -> (w1225:dbl)
            n477 = local write "MFC_1\nSLPM Value"(w1225) -> ()
            n478 = Bundle(cluster=T4 {"Message"="", "Message Data"=variant} ("Message Cluster"), "Message"="MFC_1", "Message Data"=w1225) -> (w1228:T4)
            n479 = Enqueue Element(queue=w1230, element=w1228, error in (no error)=w1229) -> (queue out=w1227:refnum<queue>, error out=w1226:errorcluster)  [unwired: 1 in, 1 out]
          }
          frame #2 {
            n480 = for {
              N: 45 -> [w1239]
              i -> [w1238]
              n481 = Subtract(x=w1239, y=w1238) -> (x-y=w1237:i32)
              n482 = Decrement(x=w1237) -> (x-1=→"Low Cal\nFlush Time Remain (sec)":i32)
              n483 = Wait (ms)(milliseconds to wait=u32 1000) -> ()  [unwired: 1 out]
            }
          }
          frame #3 {
            w1243 = TRUE
            n484 = Bundle(cluster=T4 {"Message"="", "Message Data"=variant} ("Message Cluster"), "Message"="V1", "Message Data"=w1243) -> (w1246:T4)
            n485 = local write "eV1"(w1243) -> ()
            n486 = Enqueue Element(queue=w1245, element=w1246, error in (no error)=w1244) -> (queue out=w1242:refnum<queue>, error out=w1241:errorcluster)  [unwired: 1 in, 1 out]
          }
          frame #4 {
            n487 = for {
              N: 60 -> [w1255]
              i -> [w1254]
              n488 = Subtract(x=w1255, y=w1254) -> (x-y=w1253:i32)
              n489 = Decrement(x=w1253) -> (x-1=→"Low Cal\nCal Time Remain (sec)":i32)
              n490 = Wait (ms)(milliseconds to wait=u32 1000) -> ()  [unwired: 1 out]
            }
          }
          frame #5 {
            w1259 = FALSE
            n491 = Cluster To Array(cluster=T13 {"Message"="V2", "Message 3"="V4", "Message 4"="V1"}) -> (array=w1262:string[])
            n492 = for {
              tunnel: w1262 -> [w1269] mode=indexing
              tunnel: [w1268] -> w1258
              tunnel: [w1267] -> w1257
              tunnel: w1259 -> [w1266]
              tunnel: w1261 -> [w1265]
              tunnel: w1260 -> [w1264]
              n493 = Bundle(cluster=T4 {"Message"="", "Message Data"=variant} ("Message Cluster"), "Message"=w1269, "Message Data"=w1266) -> (w1271:T4)
              n494 = Enqueue Element(queue=w1265, element=w1271, error in (no error)=w1264) -> (queue out=w1268:refnum<queue>, error out=w1267:errorcluster)  [unwired: 1 in, 1 out]
            }
            n495 = local write "eV2"(w1259) -> ()
            n496 = local write "eV4"(w1259) -> ()
            n497 = local write "eV1"(w1259) -> ()
          }
          frame #6 {
            w1273 = 0.0 ("MFC_1\nSLPM Value")
            n498 = local write "MFC_1\nSLPM Value"(w1273) -> ()
            n499 = Bundle(cluster=T4 {"Message"="", "Message Data"=variant} ("Message Cluster"), "Message"="MFC_1", "Message Data"=w1273) -> (w1277:T4)
            n500 = Enqueue Element(queue=w1275, element=w1277, error in (no error)=w1274) -> (error out=w1272:errorcluster)  [unwired: 1 in, 2 out]
          }
          frame #7 {
            n501 = local write "Low Cal"(FALSE ("High Cal")) -> ()
          }
        }
      }
      event "Target Cal": Value Change {
        n502 = event-data() -> ()  [unwired: 1 in, 1 out]
        n503 = flat-sequence {
          tunnel: w1296 -> [w1304]
          tunnel: w1295 -> [w1303]
          tunnel: [w1302] -> w1294
          tunnel: [w1301] -> w1293
          tunnel: w1294 -> [w1310]
          tunnel: w1293 -> [w1309]
          tunnel: [w1307] -> w1291
          tunnel: [w1306] -> w1289
          tunnel: [w1315] -> w1292
          tunnel: w1291 -> [w1315]
          tunnel: [w1314] -> w1290
          tunnel: w1289 -> [w1314]
          tunnel: w1292 -> [w1325]
          tunnel: w1290 -> [w1324]
          tunnel: [w1322] -> w1287
          tunnel: [w1321] -> w1285
          tunnel: [w1331] -> w1288
          tunnel: w1287 -> [w1331]
          tunnel: [w1330] -> w1286
          tunnel: w1285 -> [w1330]
          tunnel: w1288 -> [w1340]
          tunnel: w1286 -> [w1339]
          tunnel: [w1337] -> w1284
          tunnel: [w1338] -> w1283
          tunnel: w1284 -> [w1355]
          tunnel: w1283 -> [w1354]
          tunnel: [w1352] -> w1281
          tunnel: [w1360] -> w1282
          tunnel: w1281 -> [w1360]
          frame #0 {
            w1300 = TRUE
            n504 = local write "eV4"(w1300) -> ()
            n505 = Bundle(cluster=T4 {"Message"="", "Message Data"=variant} ("Message Cluster"), "Message"="V4" ("Message 3"), "Message Data"=w1300) -> (w1299:T4)
            n506 = Enqueue Element(queue=w1304, element=w1299, error in (no error)=w1303) -> (queue out=w1302:refnum<queue>, error out=w1301:errorcluster)  [unwired: 1 in, 1 out]
          }
          frame #1 {
            n507 = local read "MFC_1 User Set Value"() -> (w1305:dbl)
            n508 = local write "MFC_1\nSLPM Value"(w1305) -> ()
            n509 = Bundle(cluster=T4 {"Message"="", "Message Data"=variant} ("Message Cluster"), "Message"="MFC_1", "Message Data"=w1305) -> (w1308:T4)
            n510 = Enqueue Element(queue=w1310, element=w1308, error in (no error)=w1309) -> (queue out=w1307:refnum<queue>, error out=w1306:errorcluster)  [unwired: 1 in, 1 out]
          }
          frame #2 {
            n511 = for {
              N: 45 -> [w1319]
              i -> [w1318]
              n512 = Subtract(x=w1319, y=w1318) -> (x-y=w1317:i32)
              n513 = Decrement(x=w1317) -> (x-1=→"Target Cal\nFlush Time Remain (sec)":i32)
              n514 = Wait (ms)(milliseconds to wait=u32 1000) -> ()  [unwired: 1 out]
            }
          }
          frame #3 {
            w1323 = TRUE
            n515 = Bundle(cluster=T4 {"Message"="", "Message Data"=variant} ("Message Cluster"), "Message"="V1", "Message Data"=w1323) -> (w1326:T4)
            n516 = local write "eV1"(w1323) -> ()
            n517 = Enqueue Element(queue=w1325, element=w1326, error in (no error)=w1324) -> (queue out=w1322:refnum<queue>, error out=w1321:errorcluster)  [unwired: 1 in, 1 out]
          }
          frame #4 {
            n518 = for {
              N: 60 -> [w1335]
              i -> [w1334]
              n519 = Subtract(x=w1335, y=w1334) -> (x-y=w1333:i32)
              n520 = Decrement(x=w1333) -> (x-1=→"Target Cal\nCal Time Remain (sec)":i32)
              n521 = Wait (ms)(milliseconds to wait=u32 1000) -> ()  [unwired: 1 out]
            }
          }
          frame #5 {
            w1343 = FALSE
            n522 = Cluster To Array(cluster=cluster{"Message 3":string, "Message":string} {"Message 3"="V4", "Message"="V1"}) -> (array=w1341:string[])
            n523 = for {
              tunnel: w1341 -> [w1349] mode=indexing
              tunnel: [w1348] -> w1337
              tunnel: [w1347] -> w1338
              tunnel: w1343 -> [w1346]
              tunnel: w1340 -> [w1345]
              tunnel: w1339 -> [w1344]
              n524 = Bundle(cluster=T4 {"Message"="", "Message Data"=variant} ("Message Cluster"), "Message"=w1349, "Message Data"=w1346) -> (w1351:T4)
              n525 = Enqueue Element(queue=w1345, element=w1351, error in (no error)=w1344) -> (queue out=w1348:refnum<queue>, error out=w1347:errorcluster)  [unwired: 1 in, 1 out]
            }
            n526 = local write "eV4"(w1343) -> ()
            n527 = local write "eV1"(w1343) -> ()
          }
          frame #6 {
            w1353 = 0.0 ("MFC_1\nSLPM Value")
            n528 = local write "MFC_1\nSLPM Value"(w1353) -> ()
            n529 = Bundle(cluster=T4 {"Message"="", "Message Data"=variant} ("Message Cluster"), "Message"="MFC_1", "Message Data"=w1353) -> (w1357:T4)
            n530 = Enqueue Element(queue=w1355, element=w1357, error in (no error)=w1354) -> (error out=w1352:errorcluster)  [unwired: 1 in, 2 out]
          }
          frame #7 {
            n531 = local write "Target Cal"(FALSE ("High Cal")) -> ()
          }
        }
      }
      event "MFC_1\nSLPM Value": Value Change {
        n532 = event-data() -> ()  [unwired: 1 in, 1 out]
        n533 = local read "MFC_1\nSLPM Value"() -> (w1361:dbl)
        n534 = Bundle(cluster=T4 {"Message"="", "Message Data"=variant} ("Message Cluster"), "Message"="MFC_1", "Message Data"=w1361) -> (w1365:T4)
        n535 = Enqueue Element(queue=w1364, element=w1365, error in (no error)=w1363) -> (error out=w1362:errorcluster)  [unwired: 1 in, 2 out]
      }
      event "FGGA UDP Time Offset": Value Change {
        n536 = event-data() -> ("NewVal"=w1368:i32)  [unwired: 1 in, 5 out]
        n537 = Bundle(cluster=T4 {"Message"="", "Message Data"=variant} ("Message Cluster"), "Message"="UDP Time Offset", "Message Data"=w1368) -> (w1372:T4)
        n538 = Enqueue Element(queue=w1371, element=w1372, error in (no error)=w1370) -> (error out=w1369:errorcluster)  [unwired: 1 in, 2 out]
      }
    }
    "FGGA Event Error out" <- w663
  }
  n539 = Create Network Stream Writer Endpoint(6:w53, 7:10 ("writer buffer size"), 9:w55, 10:"//192.168.101.17/command/reader/FGGA" ("reader url"), 11:"/command/writer/FGGA" ("writer name")) -> (0:w52:errorcluster, 3:w51:refnum<k21>)  [unwired: 2 in]
  n540 = node-c288(w11) -> ()  [unwired: 1 out]
  n541 = while {
    tunnel: w2 -> [w1382]
    shift-right: [w1377] -> _
    shift-left: w51 -> [w1379]
    shift-right: [w1375] -> w48
    shift-left: w52 -> [w1381]
    tunnel: w1 -> [w1376]
    stop <- w1375 stop-if-true
    # "FGGA UI Command Sender"
    n542 = Dequeue Element(queue=w1382, error in (no error)=w1376) -> (element=w1378:T4)  [unwired: 1 in, 3 out]
    n543 = Unbundle By Name(w1378) -> ("Message"=w1380:string)
    n544 = case shown="\"UDP Time Offset\"" w1380 {
      tunnel: w1381 -> [w1383 w1387 w1394 w1401 w1408 w1415 w1422 w1429 w1436 w1443 w1450]
      tunnel: w1379 -> [w1384 w1390 w1397 w1404 w1411 w1418 w1425 w1432 w1439 w1446 w1453]
      tunnel: w1378 -> [_ w1389 w1396 w1403 w1410 w1417 w1424 w1431 w1438 w1445 w1452]
      tunnel: [w1383 w1386 w1393 w1400 w1407 w1414 w1421 w1428 w1435 w1442 w1449] -> w1375
      tunnel: [w1384 w1385 w1392 w1399 w1406 w1413 w1420 w1427 w1434 w1441 w1448] -> w1377
      frame "False", Default {
      }
      frame "V1" {
        n545 = shared-variable-write(w1390, w1387, w1389) -> (w1388:refnum<k21>, w1391:errorcluster)  [unwired: 1 in, 1 out]
        n546 = Flush Stream(8:w1391, 11:w1388) -> (0:w1386:errorcluster, 3:w1385:refnum<k21>)  [unwired: 2 in, 1 out]
      }
      frame "MFC_1" {
        n547 = shared-variable-write(w1397, w1394, w1396) -> (w1395:refnum<k21>, w1398:errorcluster)  [unwired: 1 in, 1 out]
        n548 = Flush Stream(8:w1398, 11:w1395) -> (0:w1393:errorcluster, 3:w1392:refnum<k21>)  [unwired: 2 in, 1 out]
      }
      frame "UDP Time Offset" {
        n549 = shared-variable-write(w1404, w1401, w1403) -> (w1402:refnum<k21>, w1405:errorcluster)  [unwired: 1 in, 1 out]
        n550 = Flush Stream(8:w1405, 11:w1402) -> (0:w1400:errorcluster, 3:w1399:refnum<k21>)  [unwired: 2 in, 1 out]
      }
      frame "V2" {
        n551 = shared-variable-write(w1411, w1408, w1410) -> (w1409:refnum<k21>, w1412:errorcluster)  [unwired: 1 in, 1 out]
        n552 = Flush Stream(8:w1412, 11:w1409) -> (0:w1407:errorcluster, 3:w1406:refnum<k21>)  [unwired: 2 in, 1 out]
      }
      frame "V3" {
        n553 = shared-variable-write(w1418, w1415, w1417) -> (w1416:refnum<k21>, w1419:errorcluster)  [unwired: 1 in, 1 out]
        n554 = Flush Stream(8:w1419, 11:w1416) -> (0:w1414:errorcluster, 3:w1413:refnum<k21>)  [unwired: 2 in, 1 out]
      }
      frame "V4" {
        n555 = shared-variable-write(w1425, w1422, w1424) -> (w1423:refnum<k21>, w1426:errorcluster)  [unwired: 1 in, 1 out]
        n556 = Flush Stream(8:w1426, 11:w1423) -> (0:w1421:errorcluster, 3:w1420:refnum<k21>)  [unwired: 2 in, 1 out]
      }
      frame "FGGA_pump" {
        n557 = shared-variable-write(w1432, w1429, w1431) -> (w1430:refnum<k21>, w1433:errorcluster)  [unwired: 1 in, 1 out]
        n558 = Flush Stream(8:w1433, 11:w1430) -> (0:w1428:errorcluster, 3:w1427:refnum<k21>)  [unwired: 2 in, 1 out]
      }
      frame "Flight Number" {
        n559 = shared-variable-write(w1439, w1436, w1438) -> (w1437:refnum<k21>, w1440:errorcluster)  [unwired: 1 in, 1 out]
        n560 = Flush Stream(8:w1440, 11:w1437) -> (0:w1435:errorcluster, 3:w1434:refnum<k21>)  [unwired: 2 in, 1 out]
      }
      frame "FGGA_restart" {
        n561 = shared-variable-write(w1446, w1443, w1445) -> (w1444:refnum<k21>, w1447:errorcluster)  [unwired: 1 in, 1 out]
        n562 = Flush Stream(8:w1447, 11:w1444) -> (0:w1442:errorcluster, 3:w1441:refnum<k21>)  [unwired: 2 in, 1 out]
      }
      frame "Stop File Write" {
        n563 = shared-variable-write(w1453, w1450, w1452) -> (w1451:refnum<k21>, w1454:errorcluster)  [unwired: 1 in, 1 out]
        n564 = Flush Stream(8:w1454, 11:w1451) -> (0:w1449:errorcluster, 3:w1448:refnum<k21>)  [unwired: 2 in, 1 out]
      }
    }
  }
  "FGGA command sender error out" <- w48
  n565 = Obtain Queue(name (unnamed)="SO2_Command", element data type=w37) -> (queue out=w46:refnum<queue>, error out=w39:errorcluster)  [unwired: 3 in, 1 out]
  n566 = while {
    tunnel: w46 -> [w1458]
    tunnel: w39 -> [w1457]
    tunnel: [w1455] -> _
    stop <- FALSE stop-if-true
    # "SO2 UI Event Handler Loop"
    n567 = event shown="[1] \"SO2 Flush\": Value Change" {
      selector: _ -> [_ _ _ _ _ _ _ _ _ _ _ _ _ _ _ _ _ _]
      dyn-events: _ -> [_ _ _ _ _ _ _ _ _ _ _ _ _ _ _ _ _ _]
      timeout: _ -> [_ _ _ _ _ _ _ _ _ _ _ _ _ _ _ _ _ _]
      tunnel: w1458 -> [w1465 w1477 w1526 w1565 w1634 w1641 w1645 w1652 w1659 w1666 w1673 w1680 w1687 w1694 w1701 w1708 w1715 w1722]
      tunnel: w1457 -> [w1464 w1476 w1525 w1564 w1633 w1640 w1644 w1651 w1658 w1665 w1672 w1679 w1686 w1693 w1700 w1707 w1714 w1721]
      tunnel: [w1459 w1475 w1524 _ w1628 w1635 w1643 w1650 w1657 w1664 w1671 w1678 w1685 w1692 w1699 w1706 w1713 w1720] -> w1455
      event "eV9": Value Change {
        n568 = event-data() -> ("NewVal"=w1462:bool)  [unwired: 1 in]
        n569 = Bundle(cluster=T4 {"Message"="", "Message Data"=variant} ("Message Cluster"), "Message"="V9", "Message Data"=w1462) -> (w1460:T4)
        n570 = Enqueue Element(queue=w1465, element=w1460, error in (no error)=w1464) -> (error out=w1459:errorcluster)  [unwired: 1 in, 2 out]
      }
      event "SO2 Flush": Value Change {
        n571 = event-data() -> ()  [unwired: 1 in, 1 out]
        n572 = flat-sequence {
          tunnel: w1477 -> [w1485]
          tunnel: w1476 -> [w1484]
          tunnel: [w1480] -> w1472
          tunnel: [w1478] -> w1470
          tunnel: w1472 -> [w1487]
          tunnel: [w1489] -> w1471
          tunnel: w1470 -> [w1488]
          tunnel: [w1490] -> w1469
          tunnel: w1471 -> [w1496]
          tunnel: [w1496] -> w1474
          tunnel: [w1494] -> w1473
          tunnel: w1469 -> [w1494]
          tunnel: w1474 -> [w1505]
          tunnel: [w1504] -> w1468
          tunnel: w1473 -> [w1506]
          tunnel: [w1502] -> w1466
          tunnel: w1468 -> [w1512]
          tunnel: [w1513] -> w1467
          tunnel: w1466 -> [w1511]
          tunnel: [w1518] -> w1475
          tunnel: w1467 -> [w1518]
          frame #0 {
            w1479 = TRUE ("SO2 Flush")
            n573 = Bundle(cluster=T4 {"Message"="", "Message Data"=variant} ("Message Cluster"), "Message"="V9", "Message Data"=w1479) -> (w1481:T4)
            n574 = local write "eV9"(w1479) -> ()
            n575 = Enqueue Element(queue=w1485, element=w1481, error in (no error)=w1484) -> (queue out=w1478:refnum<queue>, error out=w1480:errorcluster)  [unwired: 1 in, 1 out]
          }
          frame #1 {
            n576 = local read "MFC_2 User Set Value"() -> (w1486:dbl)
            n577 = local write "MFC_2\nSLPM Value"(w1486) -> ()
            n578 = Bundle(cluster=T4 {"Message"="", "Message Data"=variant} ("Message Cluster"), "Message"="MFC_2", "Message Data"=w1486) -> (w1491:T4)
            n579 = Enqueue Element(queue=w1488, element=w1491, error in (no error)=w1487) -> (queue out=w1490:refnum<queue>, error out=w1489:errorcluster)  [unwired: 1 in, 1 out]
          }
          frame #2 {
            n580 = for {
              N: "eV9 Flush User\nset time (sec)" -> [w1500]
              i -> [w1499]
              n581 = Subtract(x=w1500, y=w1499) -> (x-y=w1498:i32)
              n582 = Decrement(x=w1498) -> (x-1=w1497:i32)
              n583 = local write "SO2 Flush\nTime Remain (sec)"(w1497) -> ()
              n584 = Wait (ms)(milliseconds to wait=u32 1000) -> ()  [unwired: 1 out]
            }
          }
          frame #3 {
            w1503 = FALSE
            n585 = Bundle(cluster=T4 {"Message"="", "Message Data"=variant} ("Message Cluster"), "Message"="V9", "Message Data"=w1503) -> (w1507:T4)
            n586 = local write "eV9"(w1503) -> ()
            n587 = Enqueue Element(queue=w1506, element=w1507, error in (no error)=w1505) -> (queue out=w1502:refnum<queue>, error out=w1504:errorcluster)  [unwired: 1 in, 1 out]
          }
          frame #4 {
            w1510 = 0.0 ("MFC_2\nSLPM Value")
            n588 = local write "MFC_2\nSLPM Value"(w1510) -> ()
            n589 = Bundle(cluster=T4 {"Message"="", "Message Data"=variant} ("Message Cluster"), "Message"="MFC_2", "Message Data"=w1510) -> (w1514:T4)
            n590 = Enqueue Element(queue=w1511, element=w1514, error in (no error)=w1512) -> (error out=w1513:errorcluster)  [unwired: 1 in, 2 out]
          }
          frame #5 {
            n591 = local write "SO2 Flush"(FALSE ("SO2 Flush")) -> ()
          }
        }
      }
      event "SO2 Zeroing": Value Change {
        n592 = event-data() -> ()  [unwired: 1 in, 1 out]
        n593 = flat-sequence {
          tunnel: w1526 -> [w1534]
          tunnel: w1525 -> [w1533]
          tunnel: [w1529] -> w1523
          tunnel: [w1527] -> w1519
          tunnel: w1523 -> [w1537]
          tunnel: [w1537] -> w1522
          tunnel: [w1535] -> w1520
          tunnel: w1519 -> [w1535]
          tunnel: w1522 -> [w1545]
          tunnel: [w1544] -> w1521
          tunnel: w1520 -> [w1546]
          tunnel: [w1551] -> w1524
          tunnel: w1521 -> [w1551]
          frame #0 {
            w1528 = TRUE ("SO2 Flush")
            n594 = local write "SO2 eV6"(w1528) -> ()
            n595 = Bundle(cluster=T4 {"Message"="", "Message Data"=variant} ("Message Cluster"), "Message"="V6", "Message Data"=w1528) -> (w1530:T4)
            n596 = Enqueue Element(queue=w1534, element=w1530, error in (no error)=w1533) -> (queue out=w1527:refnum<queue>, error out=w1529:errorcluster)  [unwired: 1 in, 1 out]
          }
          frame #1 {
            # "10 Mins Count down"
            n597 = for {
              N: 600 -> [w1541]
              i -> [w1540]
              n598 = Subtract(x=w1541, y=w1540) -> (x-y=w1539:i32)
              n599 = Decrement(x=w1539) -> (x-1=w1538:i32)
              n600 = local write "SO2 Zeroing\nTime Remain (sec)"(w1538) -> ()
              n601 = Wait (ms)(milliseconds to wait=u32 1000) -> ()  [unwired: 1 out]
            }
          }
          frame #2 {
            w1543 = FALSE
            n602 = Bundle(cluster=T4 {"Message"="", "Message Data"=variant} ("Message Cluster"), "Message"="V6", "Message Data"=w1543) -> (w1547:T4)
            n603 = local write "SO2 eV6"(w1543) -> ()
            n604 = Enqueue Element(queue=w1546, element=w1547, error in (no error)=w1545) -> (error out=w1544:errorcluster)  [unwired: 1 in, 2 out]
          }
          frame #3 {
            n605 = local write "SO2 Zeroing"(FALSE ("SO2 Flush")) -> ()
          }
        }
      }
      event "SO2 CAL": Value Change {
        n606 = event-data() -> ()  [unwired: 1 in, 1 out]
        n607 = flat-sequence {
          tunnel: w1565 -> [w1573]
          tunnel: w1564 -> [w1572]
          tunnel: [w1568] -> w1563
          tunnel: [w1567] -> w1561
          tunnel: w1563 -> [w1577]
          tunnel: [w1576] -> w1562
          tunnel: w1561 -> [w1578]
          tunnel: [w1574] -> w1559
          tunnel: w1562 -> [w1584]
          tunnel: [w1584] -> w1560
          tunnel: w1559 -> [w1582]
          tunnel: [w1582] -> w1558
          tunnel: w1560 -> [w1593]
          tunnel: w1558 -> [w1594]
          tunnel: [w1591] -> w1556
          tunnel: [w1590] -> w1554
          tunnel: [w1599] -> w1557
          tunnel: w1556 -> [w1599]
          tunnel: [w1598] -> w1555
          tunnel: w1554 -> [w1598]
          tunnel: w1557 -> [w1609]
          tunnel: w1555 -> [w1608]
          tunnel: [w1607] -> w1553
          tunnel: [w1606] -> w1552
          tunnel: w1553 -> [w1623]
          tunnel: w1552 -> [w1622]
          frame #0 {
            w1566 = TRUE ("SO2 Flush")
            n608 = Bundle(cluster=T4 {"Message"="", "Message Data"=variant} ("Message Cluster"), "Message"="V9", "Message Data"=w1566) -> (w1569:T4)
            n609 = local write "eV9"(w1566) -> ()
            n610 = Enqueue Element(queue=w1573, element=w1569, error in (no error)=w1572) -> (queue out=w1567:refnum<queue>, error out=w1568:errorcluster)  [unwired: 1 in, 1 out]
          }
          frame #1 {
            n611 = local read "MFC_2 User Set Value"() -> (w1575:dbl)
            n612 = local write "MFC_2\nSLPM Value"(w1575) -> ()
            n613 = Bundle(cluster=T4 {"Message"="", "Message Data"=variant} ("Message Cluster"), "Message"="MFC_2", "Message Data"=w1575) -> (w1579:T4)
            n614 = Enqueue Element(queue=w1578, element=w1579, error in (no error)=w1577) -> (queue out=w1574:refnum<queue>, error out=w1576:errorcluster)  [unwired: 1 in, 1 out]
          }
          frame #2 {
            n615 = for {
              N: "eV9 flush User\nset time (sec)" -> [w1588]
              i -> [w1587]
              n616 = Subtract(x=w1588, y=w1587) -> (x-y=w1586:i32)
              n617 = Decrement(x=w1586) -> (x-1=w1585:i32)
              n618 = local write "SO2 Cal Flush\nTime Remain (sec)"(w1585) -> ()
              n619 = Wait (ms)(milliseconds to wait=u32 1000) -> ()  [unwired: 1 out]
            }
          }
          frame #3 {
            w1592 = TRUE ("SO2 Flush")
            n620 = Bundle(cluster=T4 {"Message"="", "Message Data"=variant} ("Message Cluster"), "Message"="V8", "Message Data"=w1592) -> (w1595:T4)
            n621 = local write "eV8"(w1592) -> ()
            n622 = Enqueue Element(queue=w1594, element=w1595, error in (no error)=w1593) -> (queue out=w1591:refnum<queue>, error out=w1590:errorcluster)  [unwired: 1 in, 1 out]
          }
          frame #4 {
            n623 = for {
              N: "eV8 User\nset time (sec)" -> [w1604]
              i -> [w1603]
              n624 = Subtract(x=w1604, y=w1603) -> (x-y=w1602:i32)
              n625 = Decrement(x=w1602) -> (x-1=w1601:i32)
              n626 = local write "SO2 CAL\nTime Remain (sec)"(w1601) -> ()
              n627 = Wait (ms)(milliseconds to wait=u32 1000) -> ()  [unwired: 1 out]
            }
          }
          frame #5 {
            n628 = Cluster To Array(cluster=cluster{"Message":string, "Message 2":string} {"Message"="V8", "Message 2"="V9"}) -> (array=w1611:string[])
            n629 = for {
              tunnel: w1611 -> [w1618] mode=indexing
              tunnel: FALSE ("SO2 Flush") -> [w1617]
              tunnel: w1609 -> [w1616]
              tunnel: w1608 -> [w1615]
              tunnel: [w1614] -> w1607
              tunnel: [w1613] -> w1606
              n630 = Bundle(cluster=T4 {"Message"="", "Message Data"=variant} ("Message Cluster"), "Message"=w1618, "Message Data"=w1617) -> (w1619:T4)
              n631 = Enqueue Element(queue=w1616, element=w1619, error in (no error)=w1615) -> (queue out=w1614:refnum<queue>, error out=w1613:errorcluster)  [unwired: 1 in, 1 out]
            }
          }
          frame #6 {
            w1621 = 0.0 ("MFC_2\nSLPM Value")
            n632 = local write "MFC_2\nSLPM Value"(w1621) -> ()
            n633 = Bundle(cluster=T4 {"Message"="", "Message Data"=variant} ("Message Cluster"), "Message"="MFC_2", "Message Data"=w1621) -> (w1624:T4)
            n634 = Enqueue Element(queue=w1623, element=w1624, error in (no error)=w1622) -> ()  [unwired: 1 in, 3 out]
          }
          frame #7 {
            w1627 = FALSE ("SO2 Flush")
            n635 = local write "SO2 CAL"(w1627) -> ()
            n636 = local write "eV9"(w1627) -> ()
            n637 = local write "eV8"(w1627) -> ()
          }
        }
      }
      event "MFC_2\nSLPM Value": Value Change {
        n638 = event-data() -> ("NewVal"=w1631:dbl)  [unwired: 1 in]
        n639 = Bundle(cluster=T4 {"Message"="", "Message Data"=variant} ("Message Cluster"), "Message"="MFC_2", "Message Data"=w1631) -> (w1629:T4)
        n640 = Enqueue Element(queue=w1634, element=w1629, error in (no error)=w1633) -> (error out=w1628:errorcluster)  [unwired: 1 in, 2 out]
      }
      event "MFC_3\nSLPM Value": Value Change {
        n641 = event-data() -> ("NewVal"=w1638:dbl)  [unwired: 1 in]
        n642 = Bundle(cluster=T4 {"Message"="", "Message Data"=variant} ("Message Cluster"), "Message"="MFC_3", "Message Data"=w1638) -> (w1636:T4)
        n643 = Enqueue Element(queue=w1641, element=w1636, error in (no error)=w1640) -> (error out=w1635:errorcluster)  [unwired: 1 in, 2 out]
      }
      event "eV8": Value Change {
        n644 = event-data() -> ("NewVal"=w1642:bool)  [unwired: 1 in]
        n645 = Bundle(cluster=T4 {"Message"="", "Message Data"=variant} ("Message Cluster"), "Message"="V8", "Message Data"=w1642) -> (w1646:T4)
        n646 = Enqueue Element(queue=w1645, element=w1646, error in (no error)=w1644) -> (error out=w1643:errorcluster)  [unwired: 1 in, 2 out]
      }
      event "SO2 eV6": Value Change {
        n647 = event-data() -> ("NewVal"=w1649:bool)  [unwired: 1 in]
        n648 = Bundle(cluster=T4 {"Message"="", "Message Data"=variant} ("Message Cluster"), "Message"="V6", "Message Data"=w1649) -> (w1653:T4)
        n649 = Enqueue Element(queue=w1652, element=w1653, error in (no error)=w1651) -> (error out=w1650:errorcluster)  [unwired: 1 in, 2 out]
      }
      event "Simulate Conc": Value Change {
        n650 = event-data() -> ("NewVal"=w1656:bool)  [unwired: 1 in]
        n651 = Bundle(cluster=T4 {"Message"="", "Message Data"=variant} ("Message Cluster"), "Message"="Simulate Conc", "Message Data"=w1656) -> (w1660:T4)
        n652 = Enqueue Element(queue=w1659, element=w1660, error in (no error)=w1658) -> (error out=w1657:errorcluster)  [unwired: 1 in, 2 out]
      }
      event "SO2 UDP Time Offset": Value Change {
        n653 = event-data() -> ("NewVal"=w1663:i32)  [unwired: 1 in]
        n654 = Bundle(cluster=T4 {"Message"="", "Message Data"=variant} ("Message Cluster"), "Message"="UDP Time Offset", "Message Data"=w1663) -> (w1667:T4)
        n655 = Enqueue Element(queue=w1666, element=w1667, error in (no error)=w1665) -> (error out=w1664:errorcluster)  [unwired: 1 in, 2 out]
      }
      event "Simulate STEL Conc": Value Change {
        n656 = event-data() -> ("NewVal"=w1670:dbl)  [unwired: 1 in]
        n657 = Bundle(cluster=T4 {"Message"="", "Message Data"=variant} ("Message Cluster"), "Message"="Simulate STEL Conc", "Message Data"=w1670) -> (w1674:T4)
        n658 = Enqueue Element(queue=w1673, element=w1674, error in (no error)=w1672) -> (error out=w1671:errorcluster)  [unwired: 1 in, 2 out]
      }
      event "Simulate TWA Conc": Value Change {
        n659 = event-data() -> ("NewVal"=w1677:dbl)  [unwired: 1 in]
        n660 = Bundle(cluster=T4 {"Message"="", "Message Data"=variant} ("Message Cluster"), "Message"="Simulate TWA Conc", "Message Data"=w1677) -> (w1681:T4)
        n661 = Enqueue Element(queue=w1680, element=w1681, error in (no error)=w1679) -> (error out=w1678:errorcluster)  [unwired: 1 in, 2 out]
      }
      event "10mins STEL Limit": Value Change {
        n662 = event-data() -> ("NewVal"=w1684:i32)  [unwired: 1 in]
        n663 = Bundle(cluster=T4 {"Message"="", "Message Data"=variant} ("Message Cluster"), "Message"="10mins STEL Limit", "Message Data"=w1684) -> (w1688:T4)
        n664 = Enqueue Element(queue=w1687, element=w1688, error in (no error)=w1686) -> (error out=w1685:errorcluster)  [unwired: 1 in, 2 out]
      }
      event "8hr TWA Limit": Value Change {
        n665 = event-data() -> ("NewVal"=w1691:i32)  [unwired: 1 in]
        n666 = Bundle(cluster=T4 {"Message"="", "Message Data"=variant} ("Message Cluster"), "Message"="8hr TWA Limit", "Message Data"=w1691) -> (w1695:T4)
        n667 = Enqueue Element(queue=w1694, element=w1695, error in (no error)=w1693) -> (error out=w1692:errorcluster)  [unwired: 1 in, 2 out]
      }
      event "SO2 Offset": Value Change {
        n668 = event-data() -> ("NewVal"=w1698:dbl)  [unwired: 1 in]
        n669 = Bundle(cluster=T4 {"Message"="", "Message Data"=variant} ("Message Cluster"), "Message"="Offset", "Message Data"=w1698) -> (w1702:T4)
        n670 = Enqueue Element(queue=w1701, element=w1702, error in (no error)=w1700) -> (error out=w1699:errorcluster)  [unwired: 1 in, 2 out]
      }
      event "SO2 Slope": Value Change {
        n671 = event-data() -> ("NewVal"=w1705:dbl)  [unwired: 1 in]
        n672 = Bundle(cluster=T4 {"Message"="", "Message Data"=variant} ("Message Cluster"), "Message"="Slope", "Message Data"=w1705) -> (w1709:T4)
        n673 = Enqueue Element(queue=w1708, element=w1709, error in (no error)=w1707) -> (error out=w1706:errorcluster)  [unwired: 1 in, 2 out]
      }
      event "Confirm Flight Number": Value Change {
        n674 = event-data() -> ()  [unwired: 1 in, 6 out]
        n675 = local read "Flight Number"() -> (w1712:string)
        n676 = Bundle(cluster=T4 {"Message"="", "Message Data"=variant} ("Message Cluster"), "Message"="Flight Number", "Message Data"=w1712) -> (w1716:T4)
        n677 = Enqueue Element(queue=w1715, element=w1716, error in (no error)=w1714) -> (error out=w1713:errorcluster)  [unwired: 1 in, 2 out]
      }
      event "cRIO File IO Stop\n(USB Flash Drive Unmount)": Value Change {
        n678 = event-data() -> ("NewVal"=w1719:bool)  [unwired: 1 in]
        n679 = Bundle(cluster=T4 {"Message"="", "Message Data"=variant} ("Message Cluster"), "Message"="Stop File Write", "Message Data"=w1719) -> (w1723:T4)
        n680 = Enqueue Element(queue=w1722, element=w1723, error in (no error)=w1721) -> (error out=w1720:errorcluster)  [unwired: 1 in, 2 out]
      }
    }
    "SO2 Event error out" <- w1455
  }
  n681 = Create Network Stream Writer Endpoint(6:w43, 7:10 ("writer buffer size"), 9:w37, 10:"//192.168.101.17/command/reader/SO2" ("reader url"), 11:"/command/writer/SO2" ("writer name")) -> (0:w42:errorcluster, 3:w41:refnum<k21>)  [unwired: 2 in]
  n682 = while {
    tunnel: w46 -> [w1733]
    shift-right: [w1728] -> _
    shift-left: w41 -> [w1730]
    shift-right: [w1726] -> w38
    shift-left: w42 -> [w1732]
    tunnel: w39 -> [w1727]
    stop <- w1726 stop-if-true
    # "SO2 UI Command Sender"
    n683 = Dequeue Element(queue=w1733, error in (no error)=w1727) -> (element=w1729:T4)  [unwired: 1 in, 3 out]
    n684 = Unbundle By Name(w1729) -> ("Message"=w1731:string)
    n685 = case shown="\"UDP Time Offset\"" w1731 {
      tunnel: w1732 -> [w1734 w1738 w1745 w1752 w1759 w1766 w1773 w1780 w1787 w1794 w1801 w1808 w1815 w1822 w1829 w1836]
      tunnel: w1730 -> [w1735 w1741 w1748 w1755 w1762 w1769 w1776 w1783 w1790 w1797 w1804 w1811 w1818 w1825 w1832 w1839]
      tunnel: w1729 -> [_ w1740 w1747 w1754 w1761 w1768 w1775 w1782 w1789 w1796 w1803 w1810 w1817 w1824 w1831 w1838]
      tunnel: [w1734 w1737 w1744 w1751 w1758 w1765 w1772 w1779 w1786 w1793 w1800 w1807 w1814 w1821 w1828 w1835] -> w1726
      tunnel: [w1735 w1736 w1743 w1750 w1757 w1764 w1771 w1778 w1785 w1792 w1799 w1806 w1813 w1820 w1827 w1834] -> w1728
      frame "False", Default {
      }
      frame "V9" {
        n686 = shared-variable-write(w1741, w1738, w1740) -> (w1739:refnum<k21>, w1742:errorcluster)  [unwired: 1 in, 1 out]
        n687 = Flush Stream(8:w1742, 11:w1739) -> (0:w1737:errorcluster, 3:w1736:refnum<k21>)  [unwired: 2 in, 1 out]
      }
      frame "MFC_2" {
        n688 = shared-variable-write(w1748, w1745, w1747) -> (w1746:refnum<k21>, w1749:errorcluster)  [unwired: 1 in, 1 out]
        n689 = Flush Stream(8:w1749, 11:w1746) -> (0:w1744:errorcluster, 3:w1743:refnum<k21>)  [unwired: 2 in, 1 out]
      }
      frame "MFC_3" {
        n690 = shared-variable-write(w1755, w1752, w1754) -> (w1753:refnum<k21>, w1756:errorcluster)  [unwired: 1 in, 1 out]
        n691 = Flush Stream(8:w1756, 11:w1753) -> (0:w1751:errorcluster, 3:w1750:refnum<k21>)  [unwired: 2 in, 1 out]
      }
      frame "V6" {
        n692 = shared-variable-write(w1762, w1759, w1761) -> (w1760:refnum<k21>, w1763:errorcluster)  [unwired: 1 in, 1 out]
        n693 = Flush Stream(8:w1763, 11:w1760) -> (0:w1758:errorcluster, 3:w1757:refnum<k21>)  [unwired: 2 in, 1 out]
      }
      frame "Simulate Conc" {
        n694 = shared-variable-write(w1769, w1766, w1768) -> (w1767:refnum<k21>, w1770:errorcluster)  [unwired: 1 in, 1 out]
        n695 = Flush Stream(8:w1770, 11:w1767) -> (0:w1765:errorcluster, 3:w1764:refnum<k21>)  [unwired: 2 in, 1 out]
      }
      frame "Simulate STEL Conc" {
        n696 = shared-variable-write(w1776, w1773, w1775) -> (w1774:refnum<k21>, w1777:errorcluster)  [unwired: 1 in, 1 out]
        n697 = Flush Stream(8:w1777, 11:w1774) -> (0:w1772:errorcluster, 3:w1771:refnum<k21>)  [unwired: 2 in, 1 out]
      }
      frame "Simulate TWA Conc" {
        n698 = shared-variable-write(w1783, w1780, w1782) -> (w1781:refnum<k21>, w1784:errorcluster)  [unwired: 1 in, 1 out]
        n699 = Flush Stream(8:w1784, 11:w1781) -> (0:w1779:errorcluster, 3:w1778:refnum<k21>)  [unwired: 2 in, 1 out]
      }
      frame "10mins STEL Limit" {
        n700 = shared-variable-write(w1790, w1787, w1789) -> (w1788:refnum<k21>, w1791:errorcluster)  [unwired: 1 in, 1 out]
        n701 = Flush Stream(8:w1791, 11:w1788) -> (0:w1786:errorcluster, 3:w1785:refnum<k21>)  [unwired: 2 in, 1 out]
      }
      frame "8hr TWA Limit" {
        n702 = shared-variable-write(w1797, w1794, w1796) -> (w1795:refnum<k21>, w1798:errorcluster)  [unwired: 1 in, 1 out]
        n703 = Flush Stream(8:w1798, 11:w1795) -> (0:w1793:errorcluster, 3:w1792:refnum<k21>)  [unwired: 2 in, 1 out]
      }
      frame "Offset" {
        n704 = shared-variable-write(w1804, w1801, w1803) -> (w1802:refnum<k21>, w1805:errorcluster)  [unwired: 1 in, 1 out]
        n705 = Flush Stream(8:w1805, 11:w1802) -> (0:w1800:errorcluster, 3:w1799:refnum<k21>)  [unwired: 2 in, 1 out]
      }
      frame "Slope" {
        n706 = shared-variable-write(w1811, w1808, w1810) -> (w1809:refnum<k21>, w1812:errorcluster)  [unwired: 1 in, 1 out]
        n707 = Flush Stream(8:w1812, 11:w1809) -> (0:w1807:errorcluster, 3:w1806:refnum<k21>)  [unwired: 2 in, 1 out]
      }
      frame "Flight Number" {
        n708 = shared-variable-write(w1818, w1815, w1817) -> (w1816:refnum<k21>, w1819:errorcluster)  [unwired: 1 in, 1 out]
        n709 = Flush Stream(8:w1819, 11:w1816) -> (0:w1814:errorcluster, 3:w1813:refnum<k21>)  [unwired: 2 in, 1 out]
      }
      frame "Stop File Write" {
        n710 = shared-variable-write(w1825, w1822, w1824) -> (w1823:refnum<k21>, w1826:errorcluster)  [unwired: 1 in, 1 out]
        n711 = Flush Stream(8:w1826, 11:w1823) -> (0:w1821:errorcluster, 3:w1820:refnum<k21>)  [unwired: 2 in, 1 out]
      }
      frame "UDP Time Offset" {
        n712 = shared-variable-write(w1832, w1829, w1831) -> (w1830:refnum<k21>, w1833:errorcluster)  [unwired: 1 in, 1 out]
        n713 = Flush Stream(8:w1833, 11:w1830) -> (0:w1828:errorcluster, 3:w1827:refnum<k21>)  [unwired: 2 in, 1 out]
      }
      frame "V8" {
        n714 = shared-variable-write(w1839, w1836, w1838) -> (w1837:refnum<k21>, w1840:errorcluster)  [unwired: 1 in, 1 out]
        n715 = Flush Stream(8:w1840, 11:w1837) -> (0:w1835:errorcluster, 3:w1834:refnum<k21>)  [unwired: 2 in, 1 out]
      }
    }
  }
  "SO2 command sender error out" <- w38
  n716 = Obtain Queue(name (unnamed)="TEi43c_Command", element data type=w26) -> (queue out=w35:refnum<queue>, error out=w28:errorcluster)  [unwired: 3 in, 1 out]
  n717 = Create Network Stream Writer Endpoint(6:w32, 7:10 ("writer buffer size"), 9:w26, 10:"//192.168.101.17/command/reader/TEi43c" ("reader url"), 11:"/command/writer/TEi43c" ("writer name")) -> (0:w31:errorcluster, 3:w30:refnum<k21>)  [unwired: 2 in]
  n718 = while {
    tunnel: w35 -> [w1844]
    tunnel: w28 -> [w1843]
    tunnel: [w1841] -> _
    stop <- FALSE stop-if-true
    # "TEi43c Ozone UI Event Handler Loop"
    n719 = event shown="[0] \"Ozone Zeroing\": Value Change" {
      selector: _ -> [_ _ _ _ _]
      dyn-events: _ -> [_ _ _ _ _]
      timeout: _ -> [_ _ _ _ _]
      tunnel: w1844 -> [w1852 w1880 w1888 w1895 w1902]
      tunnel: w1843 -> [w1851 w1879 w1887 w1894 w1901]
      tunnel: [w1850 w1878 w1886 w1893 w1900] -> w1841
      event "Ozone Zeroing": Value Change {
        n720 = event-data() -> ()  [unwired: 1 in, 6 out]
        n721 = flat-sequence {
          tunnel: w1852 -> [w1857]
          tunnel: w1851 -> [w1856]
          tunnel: [w1855] -> w1849
          tunnel: [w1853] -> w1845
          tunnel: w1849 -> [w1863]
          tunnel: [w1863] -> w1848
          tunnel: [w1861] -> w1846
          tunnel: w1845 -> [w1861]
          tunnel: w1848 -> [w1871]
          tunnel: [w1870] -> w1847
          tunnel: w1846 -> [w1872]
          tunnel: [w1877] -> w1850
          tunnel: w1847 -> [w1877]
          frame #0 {
            w1854 = TRUE
            n722 = local write "Ozone eV6"(w1854) -> ()
            n723 = Bundle(cluster=T4 {"Message"="", "Message Data"=variant} ("Message Cluster"), "Message"="V6", "Message Data"=w1854) -> (w1858:T4)
            n724 = Enqueue Element(queue=w1857, element=w1858, error in (no error)=w1856) -> (queue out=w1853:refnum<queue>, error out=w1855:errorcluster)  [unwired: 1 in, 1 out]
          }
          frame #1 {
            # "10 Mins Count down"
            n725 = for {
              N: 600 -> [w1867]
              i -> [w1866]
              n726 = Subtract(x=w1867, y=w1866) -> (x-y=w1865:i32)
              n727 = Decrement(x=w1865) -> (x-1=→"Ozone Zeroing\nTime Remain (sec)":i32)
              n728 = Wait (ms)(milliseconds to wait=u32 1000) -> ()  [unwired: 1 out]
            }
          }
          frame #2 {
            w1869 = FALSE
            n729 = local write "Ozone eV6"(w1869) -> ()
            n730 = Bundle(cluster=T4 {"Message"="", "Message Data"=variant} ("Message Cluster"), "Message"="V6", "Message Data"=w1869) -> (w1873:T4)
            n731 = Enqueue Element(queue=w1872, element=w1873, error in (no error)=w1871) -> (error out=w1870:errorcluster)  [unwired: 1 in, 2 out]
          }
          frame #3 {
            n732 = local write "Ozone Zeroing"(FALSE ("Ozone Zeroing")) -> ()
          }
        }
      }
      event "Ozone eV6": Value Change {
        n733 = event-data() -> ("NewVal"=w1881:bool)  [unwired: 1 in]
        n734 = Bundle(cluster=T4 {"Message"="", "Message Data"=variant} ("Message Cluster"), "Message"="V6", "Message Data"=w1881) -> (w1882:T4)
        n735 = Enqueue Element(queue=w1880, element=w1882, error in (no error)=w1879) -> (error out=w1878:errorcluster)  [unwired: 1 in, 2 out]
      }
      event "cRIO File IO Stop\n(USB Flash Drive Unmount)": Value Change {
        n736 = event-data() -> ("NewVal"=w1885:bool)  [unwired: 1 in]
        n737 = Bundle(cluster=T4 {"Message"="", "Message Data"=variant} ("Message Cluster"), "Message"="Stop File Write", "Message Data"=w1885) -> (w1889:T4)
        n738 = Enqueue Element(queue=w1888, element=w1889, error in (no error)=w1887) -> (error out=w1886:errorcluster)  [unwired: 1 in, 2 out]
      }
      event "Ozone UDP Time Offset": Value Change {
        n739 = event-data() -> ("NewVal"=w1892:i32)  [unwired: 1 in]
        n740 = Bundle(cluster=T4 {"Message"="", "Message Data"=variant} ("Message Cluster"), "Message"="UDP Time Offset", "Message Data"=w1892) -> (w1896:T4)
        n741 = Enqueue Element(queue=w1895, element=w1896, error in (no error)=w1894) -> (error out=w1893:errorcluster)  [unwired: 1 in, 2 out]
      }
      event "Confirm Flight Number": Value Change {
        n742 = event-data() -> ()  [unwired: 1 in, 5 out]
        n743 = local read "Flight Number"() -> (w1899:string)
        n744 = Bundle(cluster=T4 {"Message"="", "Message Data"=variant} ("Message Cluster"), "Message"="Flight Number", "Message Data"=w1899) -> (w1903:T4)
        n745 = Enqueue Element(queue=w1902, element=w1903, error in (no error)=w1901) -> (error out=w1900:errorcluster)  [unwired: 1 in, 2 out]
      }
    }
    "Ozone Event error out" <- w1841
  }
  n746 = while {
    tunnel: w35 -> [w1913]
    shift-right: [w1908] -> _
    shift-left: w30 -> [w1910]
    shift-right: [w1906] -> w27
    shift-left: w31 -> [w1912]
    tunnel: w28 -> [w1907]
    stop <- w1906 stop-if-true
    # "TEi43c Ozone UI Command Sender"
    n747 = Dequeue Element(queue=w1913, error in (no error)=w1907) -> (element=w1909:T4)  [unwired: 1 in, 3 out]
    n748 = Unbundle By Name(w1909) -> ("Message"=w1911:string)
    n749 = case shown="\"UDP Time Offset\"" w1911 {
      tunnel: w1912 -> [w1914 w1918 w1925 w1932 w1939]
      tunnel: w1910 -> [w1915 w1921 w1928 w1935 w1942]
      tunnel: w1909 -> [_ w1920 w1927 w1934 w1941]
      tunnel: [w1914 w1917 w1924 w1931 w1938] -> w1906
      tunnel: [w1915 w1916 w1923 w1930 w1937] -> w1908
      frame "False", Default {
      }
      frame "V6" {
        n750 = shared-variable-write(w1921, w1918, w1920) -> (w1919:refnum<k21>, w1922:errorcluster)  [unwired: 1 in, 1 out]
        n751 = Flush Stream(8:w1922, 11:w1919) -> (0:w1917:errorcluster, 3:w1916:refnum<k21>)  [unwired: 2 in, 1 out]
      }
      frame "Stop File Write" {
        n752 = shared-variable-write(w1928, w1925, w1927) -> (w1926:refnum<k21>, w1929:errorcluster)  [unwired: 1 in, 1 out]
        n753 = Flush Stream(8:w1929, 11:w1926) -> (0:w1924:errorcluster, 3:w1923:refnum<k21>)  [unwired: 2 in, 1 out]
      }
      frame "Flight Number" {
        n754 = shared-variable-write(w1935, w1932, w1934) -> (w1933:refnum<k21>, w1936:errorcluster)  [unwired: 1 in, 1 out]
        n755 = Flush Stream(8:w1936, 11:w1933) -> (0:w1931:errorcluster, 3:w1930:refnum<k21>)  [unwired: 2 in, 1 out]
      }
      frame "UDP Time Offset" {
        n756 = shared-variable-write(w1942, w1939, w1941) -> (w1940:refnum<k21>, w1943:errorcluster)  [unwired: 1 in, 1 out]
        n757 = Flush Stream(8:w1943, 11:w1940) -> (0:w1938:errorcluster, 3:w1937:refnum<k21>)  [unwired: 2 in, 1 out]
      }
    }
  }
  "Ozone command sender error out" <- w27
  n758 = Obtain Queue(name (unnamed)="2BOzone_Command", element data type=w14) -> (queue out=w23:refnum<queue>, error out=w16:errorcluster)  [unwired: 3 in, 1 out]
  n759 = Create Network Stream Writer Endpoint(6:w20, 7:10 ("writer buffer size"), 9:w14, 10:"//192.168.101.17/command/reader/2BOzone" ("reader url"), 11:"/command/writer/2BOzone" ("writer name")) -> (0:w19:errorcluster, 3:w18:refnum<k21>)  [unwired: 2 in]
  n760 = while {
    tunnel: w23 -> [w1947]
    tunnel: w16 -> [w1946]
    tunnel: [w1944] -> _
    stop <- FALSE stop-if-true
    # "2BOzone UI Event Handler Loop"
    n761 = event shown="[7] \"Confirm Flight Number\": Value Change" {
      selector: _ -> [_ _ _ _ _ _ _ _]
      dyn-events: _ -> [_ _ _ _ _ _ _ _]
      timeout: _ -> [_ _ _ _ _ _ _ _]
      tunnel: w1947 -> [w1951 w1958 w1965 w1972 w1979 w1986 w1993 w2000]
      tunnel: w1946 -> [w1950 w1957 w1964 w1971 w1978 w1985 w1992 w1999]
      tunnel: [w1949 w1956 w1963 w1970 w1977 w1984 w1991 w1998] -> w1944
      event "Ambient = OFF\nCabin = ON": Value Change {
        n762 = event-data() -> ("NewVal"=w1948:bool)  [unwired: 1 in]
        n763 = Bundle(cluster=T4 {"Message"="", "Message Data"=variant} ("Message Cluster"), "Message"="Ambient/Cabin", "Message Data"=w1948) -> (w1952:T4)
        n764 = Enqueue Element(queue=w1951, element=w1952, error in (no error)=w1950) -> (error out=w1949:errorcluster)  [unwired: 1 in, 2 out]
      }
      event "Simulate 2B Conc": Value Change {
        n765 = event-data() -> ("NewVal"=w1955:bool)  [unwired: 1 in]
        n766 = Bundle(cluster=T4 {"Message"="", "Message Data"=variant} ("Message Cluster"), "Message"="Simulate_conc", "Message Data"=w1955) -> (w1959:T4)
        n767 = Enqueue Element(queue=w1958, element=w1959, error in (no error)=w1957) -> (error out=w1956:errorcluster)  [unwired: 1 in, 2 out]
      }
      event "Simulate Inst Conc": Value Change {
        n768 = event-data() -> ("NewVal"=w1962:i32)  [unwired: 1 in]
        n769 = Bundle(cluster=T4 {"Message"="", "Message Data"=variant} ("Message Cluster"), "Message"="Simulate_inst_conc", "Message Data"=w1962) -> (w1966:T4)
        n770 = Enqueue Element(queue=w1965, element=w1966, error in (no error)=w1964) -> (error out=w1963:errorcluster)  [unwired: 1 in, 2 out]
      }
      event "Inst_alm_thresh": Value Change {
        n771 = event-data() -> ("NewVal"=w1969:i32)  [unwired: 1 in]
        n772 = Bundle(cluster=T4 {"Message"="", "Message Data"=variant} ("Message Cluster"), "Message"="Inst_alm_thresh", "Message Data"=w1969) -> (w1973:T4)
        n773 = Enqueue Element(queue=w1972, element=w1973, error in (no error)=w1971) -> (error out=w1970:errorcluster)  [unwired: 1 in, 2 out]
      }
      event "3hr_alm_thresh": Value Change {
        n774 = event-data() -> ("NewVal"=w1976:i32)  [unwired: 1 in]
        n775 = Bundle(cluster=T4 {"Message"="", "Message Data"=variant} ("Message Cluster"), "Message"="3hr_alm_thresh", "Message Data"=w1976) -> (w1980:T4)
        n776 = Enqueue Element(queue=w1979, element=w1980, error in (no error)=w1978) -> (error out=w1977:errorcluster)  [unwired: 1 in, 2 out]
      }
      event "Simulate 3hr Average Conc": Value Change {
        n777 = event-data() -> ("NewVal"=w1983:dbl)  [unwired: 1 in]
        n778 = Bundle(cluster=T4 {"Message"="", "Message Data"=variant} ("Message Cluster"), "Message"="Simulate_3hr_av_conc", "Message Data"=w1983) -> (w1987:T4)
        n779 = Enqueue Element(queue=w1986, element=w1987, error in (no error)=w1985) -> (error out=w1984:errorcluster)  [unwired: 1 in, 2 out]
      }
      event "cRIO File IO Stop\n(USB Flash Drive Unmount)": Value Change {
        n780 = event-data() -> ("NewVal"=w1990:bool)  [unwired: 1 in]
        n781 = Bundle(cluster=T4 {"Message"="", "Message Data"=variant} ("Message Cluster"), "Message"="Stop File Write", "Message Data"=w1990) -> (w1994:T4)
        n782 = Enqueue Element(queue=w1993, element=w1994, error in (no error)=w1992) -> (error out=w1991:errorcluster)  [unwired: 1 in, 2 out]
      }
      event "Confirm Flight Number": Value Change {
        n783 = event-data() -> ()  [unwired: 1 in, 5 out]
        n784 = local read "Flight Number"() -> (w1997:string)
        n785 = Bundle(cluster=T4 {"Message"="", "Message Data"=variant} ("Message Cluster"), "Message"="Flight Number", "Message Data"=w1997) -> (w2001:T4)
        n786 = Enqueue Element(queue=w2000, element=w2001, error in (no error)=w1999) -> (error out=w1998:errorcluster)  [unwired: 1 in, 2 out]
      }
    }
    "2BOzone Event error out" <- w1944
  }
  n787 = while {
    tunnel: w23 -> [w2011]
    shift-right: [w2006] -> _
    shift-left: w18 -> [w2008]
    shift-right: [w2004] -> w15
    shift-left: w19 -> [w2010]
    tunnel: w16 -> [w2005]
    stop <- w2004 stop-if-true
    # "2BOzone UI Command Sender"
    n788 = Dequeue Element(queue=w2011, error in (no error)=w2005) -> (element=w2007:T4)  [unwired: 1 in, 3 out]
    n789 = Unbundle By Name(w2007) -> ("Message"=w2009:string)
    n790 = case shown="\"3hr_alm_thresh\"" w2009 {
      tunnel: w2010 -> [w2012 w2016 w2023 w2030 w2037 w2044 w2051 w2058 w2065]
      tunnel: w2008 -> [w2013 w2019 w2026 w2033 w2040 w2047 w2054 w2061 w2068]
      tunnel: w2007 -> [_ w2018 w2025 w2032 w2039 w2046 w2053 w2060 w2067]
      tunnel: [w2012 w2015 w2022 w2029 w2036 w2043 w2050 w2057 w2064] -> w2004
      tunnel: [w2013 w2014 w2021 w2028 w2035 w2042 w2049 w2056 w2063] -> w2006
      frame "False", Default {
      }
      frame "Ambient/Cabin" {
        n791 = shared-variable-write(w2019, w2016, w2018) -> (w2017:refnum<k21>, w2020:errorcluster)  [unwired: 1 in, 1 out]
        n792 = Flush Stream(8:w2020, 11:w2017) -> (0:w2015:errorcluster, 3:w2014:refnum<k21>)  [unwired: 2 in, 1 out]
      }
      frame "Simulate_conc" {
        n793 = shared-variable-write(w2026, w2023, w2025) -> (w2024:refnum<k21>, w2027:errorcluster)  [unwired: 1 in, 1 out]
        n794 = Flush Stream(8:w2027, 11:w2024) -> (0:w2022:errorcluster, 3:w2021:refnum<k21>)  [unwired: 2 in, 1 out]
      }
      frame "Simulate_inst_conc" {
        n795 = shared-variable-write(w2033, w2030, w2032) -> (w2031:refnum<k21>, w2034:errorcluster)  [unwired: 1 in, 1 out]
        n796 = Flush Stream(8:w2034, 11:w2031) -> (0:w2029:errorcluster, 3:w2028:refnum<k21>)  [unwired: 2 in, 1 out]
      }
      frame "Inst_alm_thresh" {
        n797 = shared-variable-write(w2040, w2037, w2039) -> (w2038:refnum<k21>, w2041:errorcluster)  [unwired: 1 in, 1 out]
        n798 = Flush Stream(8:w2041, 11:w2038) -> (0:w2036:errorcluster, 3:w2035:refnum<k21>)  [unwired: 2 in, 1 out]
      }
      frame "3hr_alm_thresh" {
        n799 = shared-variable-write(w2047, w2044, w2046) -> (w2045:refnum<k21>, w2048:errorcluster)  [unwired: 1 in, 1 out]
        n800 = Flush Stream(8:w2048, 11:w2045) -> (0:w2043:errorcluster, 3:w2042:refnum<k21>)  [unwired: 2 in, 1 out]
      }
      frame "Simulate_3hr_av_conc" {
        n801 = shared-variable-write(w2054, w2051, w2053) -> (w2052:refnum<k21>, w2055:errorcluster)  [unwired: 1 in, 1 out]
        n802 = Flush Stream(8:w2055, 11:w2052) -> (0:w2050:errorcluster, 3:w2049:refnum<k21>)  [unwired: 2 in, 1 out]
      }
      frame "Stop File Write" {
        n803 = shared-variable-write(w2061, w2058, w2060) -> (w2059:refnum<k21>, w2062:errorcluster)  [unwired: 1 in, 1 out]
        n804 = Flush Stream(8:w2062, 11:w2059) -> (0:w2057:errorcluster, 3:w2056:refnum<k21>)  [unwired: 2 in, 1 out]
      }
      frame "Flight Number" {
        n805 = shared-variable-write(w2068, w2065, w2067) -> (w2066:refnum<k21>, w2069:errorcluster)  [unwired: 1 in, 1 out]
        n806 = Flush Stream(8:w2069, 11:w2066) -> (0:w2064:errorcluster, 3:w2063:refnum<k21>)  [unwired: 2 in, 1 out]
      }
    }
  }
  "2BOzone command sender error out" <- w15
